vi "Main.vi"(11 "Module Admin":refnum<class "Delacor_lib_QMH_Cloneable Module Admin.lvclass">) -> ()   [LabVIEW 2020, in "NI DAQ.lvlib"]
doc: "This template is based off of the Queued Message Handler design pattern and the Queued Message Handler project template that ships with LabVIEW.\n\nThe main difference is that the queue is private to this module and communication between modules is performed via Broadcast and Request events.\n\nRequest events are wrapped in public API methods and are handled in the Event Handling Loop (EHL) of this VI. Any module can register for Broadcast events sent by this module. The EHL generates messages based on user interface actions.\n\nThe Message Handling Loop (MHL) processes messages generated by the EHL, or by other messages. The messages are string values, so new messages can be added easily to the Message Cases case structure in the MHL. Each message cluster can also provide an optional value for Message Data, which is a variant that can be converted to whatever message-specific data is required.\n_____\nBased on DQMH Project Template 6.1.0.94."
uses:
  NI DAQ.lvlib
  <vilib>/Delacor/Delacor QMH/Libraries/Cloneable Module Admin_class/Delacor_lib_QMH_Cloneable Module Admin.lvclass
  C:/Program Files (x86)/National Instruments/LabVIEW 2020/vi.lib/Delacor/Delacor QMH/Libraries/Module Admin_class/Delacor_lib_QMH_Module Admin.lvclass
  Module Data--cluster.ctl
  Support/Continuous aquisition params.ctl
  Support/Task list.ctl
  <vilib>/Delacor/Delacor QMH/Libraries/Message Queue_class/Delacor_lib_QMH_Message Queue.lvclass/Delacor_lib_QMH_Message Queue.ctl
  <vilib>/Delacor/Delacor QMH/Libraries/Cloneable Module Admin_class/Delacor_lib_QMH_Cloneable Module Admin.lvclass/Delacor_lib_QMH_Cloneable Module Admin.ctl
  Stop Argument--cluster.ctl
  <vilib>/Delacor/Delacor QMH/Libraries/Module Admin_class/Delacor_lib_QMH_Module Admin.lvclass/Delacor_lib_QMH_Module Admin.ctl
  Set device ID Argument--cluster.ctl
  Get channel list Argument--cluster.ctl
  Get channel list (Reply Payload)--cluster.ctl
  Create DO task Argument--cluster.ctl
  Create DO task (Reply Payload)--cluster.ctl
  Start task Argument--cluster.ctl
  Stop task Argument--cluster.ctl
  Write DO Argument--cluster.ctl
  Create DI channel Argument--cluster.ctl
  Read DI Argument--cluster.ctl
  Read DI (Reply Payload)--cluster.ctl
  Get task ref Argument--cluster.ctl
  Get task ref (Reply Payload)--cluster.ctl
  Create AI channel Argument--cluster.ctl
  Read AI Argument--cluster.ctl
  Read AI (Reply Payload)--cluster.ctl
  Create AO channel Argument--cluster.ctl
  AI config parameters--cluster.ctl
  Write AO Argument--cluster.ctl
  Validate connection Argument--cluster.ctl
  Validate connection (Reply Payload)--cluster.ctl
  Start continous acquisition Argument--cluster.ctl
  Stop continuous acquisition Argument--cluster.ctl
  <vilib>/Utility/miscctls.llb/LVPointTypeDef.ctl
  <vilib>/DAQmx/write.llb/DAQmx Write (Digital Bool 1Line 1Point).vi
  <vilib>/DAQmx/write.llb/DAQmx Write (Digital 1D Bool NChan 1Samp 1Line).vi
  <vilib>/DAQmx/read.llb/DAQmx Read (Digital 1D Bool 1Chan 1Samp).vi
  <vilib>/DAQmx/read.llb/DAQmx Read (Digital 1D Bool NChan 1Samp 1Line).vi
  <vilib>/DAQmx/write.llb/DAQmx Write (Analog DBL 1Chan 1Samp).vi
  <vilib>/DAQmx/write.llb/DAQmx Write (Analog 1D DBL NChan 1Samp).vi
  <vilib>/DAQmx/read.llb/DAQmx Read (Analog DBL 1Chan 1Samp).vi
  <vilib>/DAQmx/read.llb/DAQmx Read (Analog 1D DBL NChan 1Samp).vi
  <vilib>/Delacor/Delacor QMH/Libraries/Message Queue_class/Delacor_lib_QMH_Enqueue Message (Single).vi
  <vilib>/Delacor/Delacor QMH/Libraries/Cloneable Module Admin_class/Delacor_lib_QMH_Get Module ID.vi
  <vilib>/Delacor/Delacor QMH/Libraries/Module Admin_class/Delacor_lib_QMH_Get External Launch.vi
  <vilib>/DAQmx/write.llb/DAQmx Write (Digital 1D Bool 1Chan 1Samp).vi
  <vilib>/DAQmx/read.llb/DAQmx Read (Digital Bool 1Line 1Point).vi
  <vilib>/DAQmx/read.llb/DAQmx Read (Digital 1D U8 1Chan NSamp).vi
  <vilib>/DAQmx/miscellaneous.llb/DAQmx Fill In Error Info.vi
  <vilib>/Utility/error.llb/Error Cluster From Error Code.vi
  <vilib>/DAQmx/create/channels.llb/DAQmx Create Channel (DO-Digital Output).vi
  <vilib>/DAQmx/create/channels.llb/DAQmx Create Channel (DI-Digital Input).vi
  <vilib>/DAQmx/create/channels.llb/DAQmx Create Channel (AI-Voltage-Basic).vi
  <vilib>/DAQmx/create/channels.llb/DAQmx Create Channel (AO-Voltage-Basic).vi
  <vilib>/ErrorRing/Error Ring.xnode
  <vilib>/Delacor/Delacor QMH/Libraries/Message Queue_class/Delacor_lib_QMH_Message Queue.lvclass
  <resource>/objmgr/daqmx.rc
panel:
  out "error out":errorcluster
  out "Status":string
  in  "Simulate EHL Error":bool
  in  "Simulate MHL Error":bool
  # "Other QMH Modules communicate with this Module via its Public API (wrappers for its Request Events).\n\nThis Module communicates with other Modules via its Broadcast Events.\nAny module that wants to get these messages, just registers for this module's Broadcast events."
  # "This template is for the Delacor Modified Queued Message Handler design pattern.\n\nSee the block diagram for more information on how to use this template."
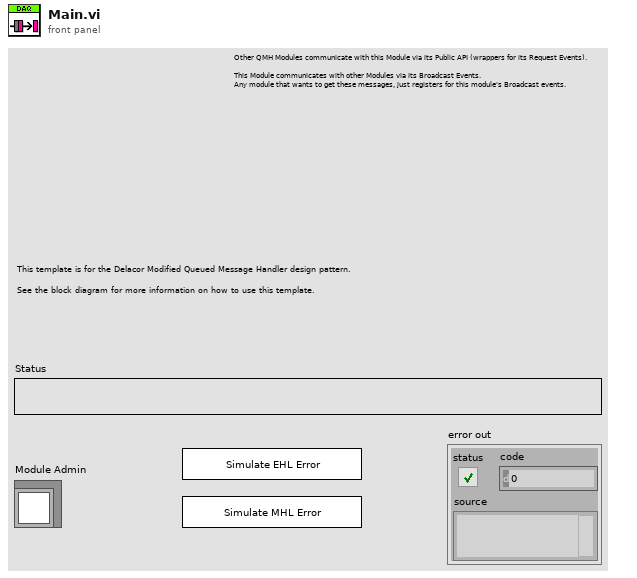
[diagram p1: front panel]
types:
  T1 = typedef "NI DAQ.lvlib/Request Events--cluster.ctl" = cluster{"Stop Module":refnum<user-event>, "Show Panel":refnum<user-event>, "Hide Panel":refnum<user-event>, "Show Diagram":refnum<user-event>, "Get Module Execution Status":refnum<user-event>, "Set device ID":refnum<user-event>, "Get channel list":refnum<user-event>, "Create DO task":refnum<user-event>, "Start task":refnum<user-event>, "Stop task":refnum<user-event>, "Write DO":refnum<user-event>, "Create DI channel":refnum<user-event>, "Read DI":refnum<user-event>, "Get task ref":refnum<user-event>, "Wake up HL":refnum<user-event>, "Sleep HL":refnum<user-event>, "Create AI channel":refnum<user-event>, "Read AI":refnum<user-event>, "Create AO channel":refnum<user-event>, "Write AO":refnum<user-event>, "Validate connection":refnum<user-event>, "Start continous acquisition":refnum<user-event>, "Stop continuous acquisition":refnum<user-event>}
  T2 = cluster{"Wake HL":refnum<user-event>, "Sleep HL":refnum<user-event>}
  T3 = typedef "NI DAQ.lvlib/Continuous aquisition params.ctl" = cluster{"Module ID":i32, "Task list":T4, "Timeout":i32, "Acq type":enum16{"Single", "Multiple"}, "Data in":variant, "DAQmx Task":refnum<k21>, "N samples":i32}
  T4 = typedef "NI DAQ.lvlib/Task list.ctl" = enum16{"All", "DO task", "DI task", "AO task", "AI task"}
  T5 = typedef "NI DAQ.lvlib/Module Data--cluster.ctl" = cluster{"Status":string, "DO task":refnum<k21>, "DI task":refnum<k21>, "AO task":refnum<k21>, "AI task":refnum<k21>, "Device name":tag}
  T6 = enum32{"invalid lock state", "Not Locked", "Locked (No Password)", "Password-protected"}
  T7 = typedef "NI DAQ.lvlib/Stop Argument--cluster.ctl" = cluster{"Module ID":i32, "Origin":string, "Exit via Stop Module Req?":bool, "Wait for Module to stop?":bool}
  T8 = typedef "NI DAQ.lvlib/Set device ID Argument--cluster.ctl" = cluster{"Module ID":i32, "Device ID":tag}
  T9 = typedef "NI DAQ.lvlib/Get channel list Argument--cluster.ctl" = cluster{"Module ID":i32, "Wait Notifier":refnum<notifier>, "wait for reply":bool}
  T10 = typedef "NI DAQ.lvlib/Create DO task Argument--cluster.ctl" = cluster{"Module ID":i32, "lines":tag, "Wait Notifier":refnum<notifier>, "wait for reply":bool, "Channel name":string}
  T11 = typedef "NI DAQ.lvlib/Start task Argument--cluster.ctl" = cluster{"Module ID":i32, "Boolean":bool}
  T12 = typedef "NI DAQ.lvlib/Stop task Argument--cluster.ctl" = cluster{"Module ID":i32, "Task list":T4}
  T13 = typedef "NI DAQ.lvlib/Write DO Argument--cluster.ctl" = cluster{"Module ID":i32, "Samples":enum16{"Single", "Multiple"}, "Data":bool[]}
  T14 = typedef "NI DAQ.lvlib/Create DI channel Argument--cluster.ctl" = cluster{"Module ID":i32, "Physical channel":string, "Channel name":string}
  T15 = typedef "NI DAQ.lvlib/Read DI Argument--cluster.ctl" = cluster{"Module ID":i32, "Samples":enum16{"Single", "Multiple"}, "Wait Notifier":refnum<notifier>, "wait for reply":bool}
  T16 = typedef "NI DAQ.lvlib/Get task ref Argument--cluster.ctl" = cluster{"Module ID":i32, "Task list":T4, "Wait Notifier":refnum<notifier>, "wait for reply":bool}
  T17 = typedef "NI DAQ.lvlib/Create AI channel Argument--cluster.ctl" = cluster{"Module ID":i32, "Physical channel":string, "Channel name":string, "Config params":cluster{"input terminal configuration":i32, "minimum value":dbl, "maximum value":dbl}}
  T18 = typedef "NI DAQ.lvlib/Read AI Argument--cluster.ctl" = cluster{"Module ID":i32, "Samples":enum16{"Single", "Multiple"}, "Wait Notifier":refnum<notifier>, "wait for reply":bool}
  T19 = typedef "NI DAQ.lvlib/Create AO channel Argument--cluster.ctl" = cluster{"Module ID":i32, "Physical channel":string, "Channel name":string, "Config params":T20}
  T20 = typedef "NI DAQ.lvlib/AI config parameters--cluster.ctl" = cluster{"Terminal configuration":i32, "min value":dbl, "max value":dbl}
  T21 = typedef "NI DAQ.lvlib/Write AO Argument--cluster.ctl" = cluster{"Module ID":i32, "Value(s)":dbl[], "Samples":enum16{"Single", "Multiple"}}
  T22 = typedef "NI DAQ.lvlib/Validate connection Argument--cluster.ctl" = cluster{"Module ID":i32, "Wait Notifier":refnum<notifier>, "wait for reply":bool}
  T23 = typedef "NI DAQ.lvlib/Start continous acquisition Argument--cluster.ctl" = cluster{"Module ID":i32, "Task list":T4, "Timeout":i32, "Acq type":enum16{"Single", "Multiple"}, "N samples":i32, "Data in":variant}
  T24 = typedef "NI DAQ.lvlib/Stop continuous acquisition Argument--cluster.ctl" = cluster{"Module ID":i32, "Boolean":bool}
  T25 = typedef "LVPointTypeDef.ctl" = cluster{"Horizontal":i16, "Vertical":i16}
  T26 = enum32{"Invalid", "Standard", "Closed", "Hidden", "Minimized", "Maximized"}
  T27 = typedef "NI DAQ.lvlib/Get channel list (Reply Payload)--cluster.ctl" = cluster{"Available channels":i32, "error":errorcluster}
  T28 = typedef "NI DAQ.lvlib/Create DO task (Reply Payload)--cluster.ctl" = cluster{"task out":refnum<k21>, "error":errorcluster}
  T29 = typedef "NI DAQ.lvlib/Read DI (Reply Payload)--cluster.ctl" = cluster{"Data":bool[], "error":errorcluster}
  T30 = typedef "NI DAQ.lvlib/Read AI (Reply Payload)--cluster.ctl" = cluster{"Data":dbl[], "error":errorcluster}
  T31 = typedef "NI DAQ.lvlib/Get task ref (Reply Payload)--cluster.ctl" = cluster{"DAQmx Task":refnum<k21>, "error":errorcluster}
  T32 = typedef "NI DAQ.lvlib/Validate connection (Reply Payload)--cluster.ctl" = cluster{"DevSerialNum":u32, "error":errorcluster}
  T33 = cluster{"input terminal configuration":i32, "minimum value":dbl, "maximum value":dbl}
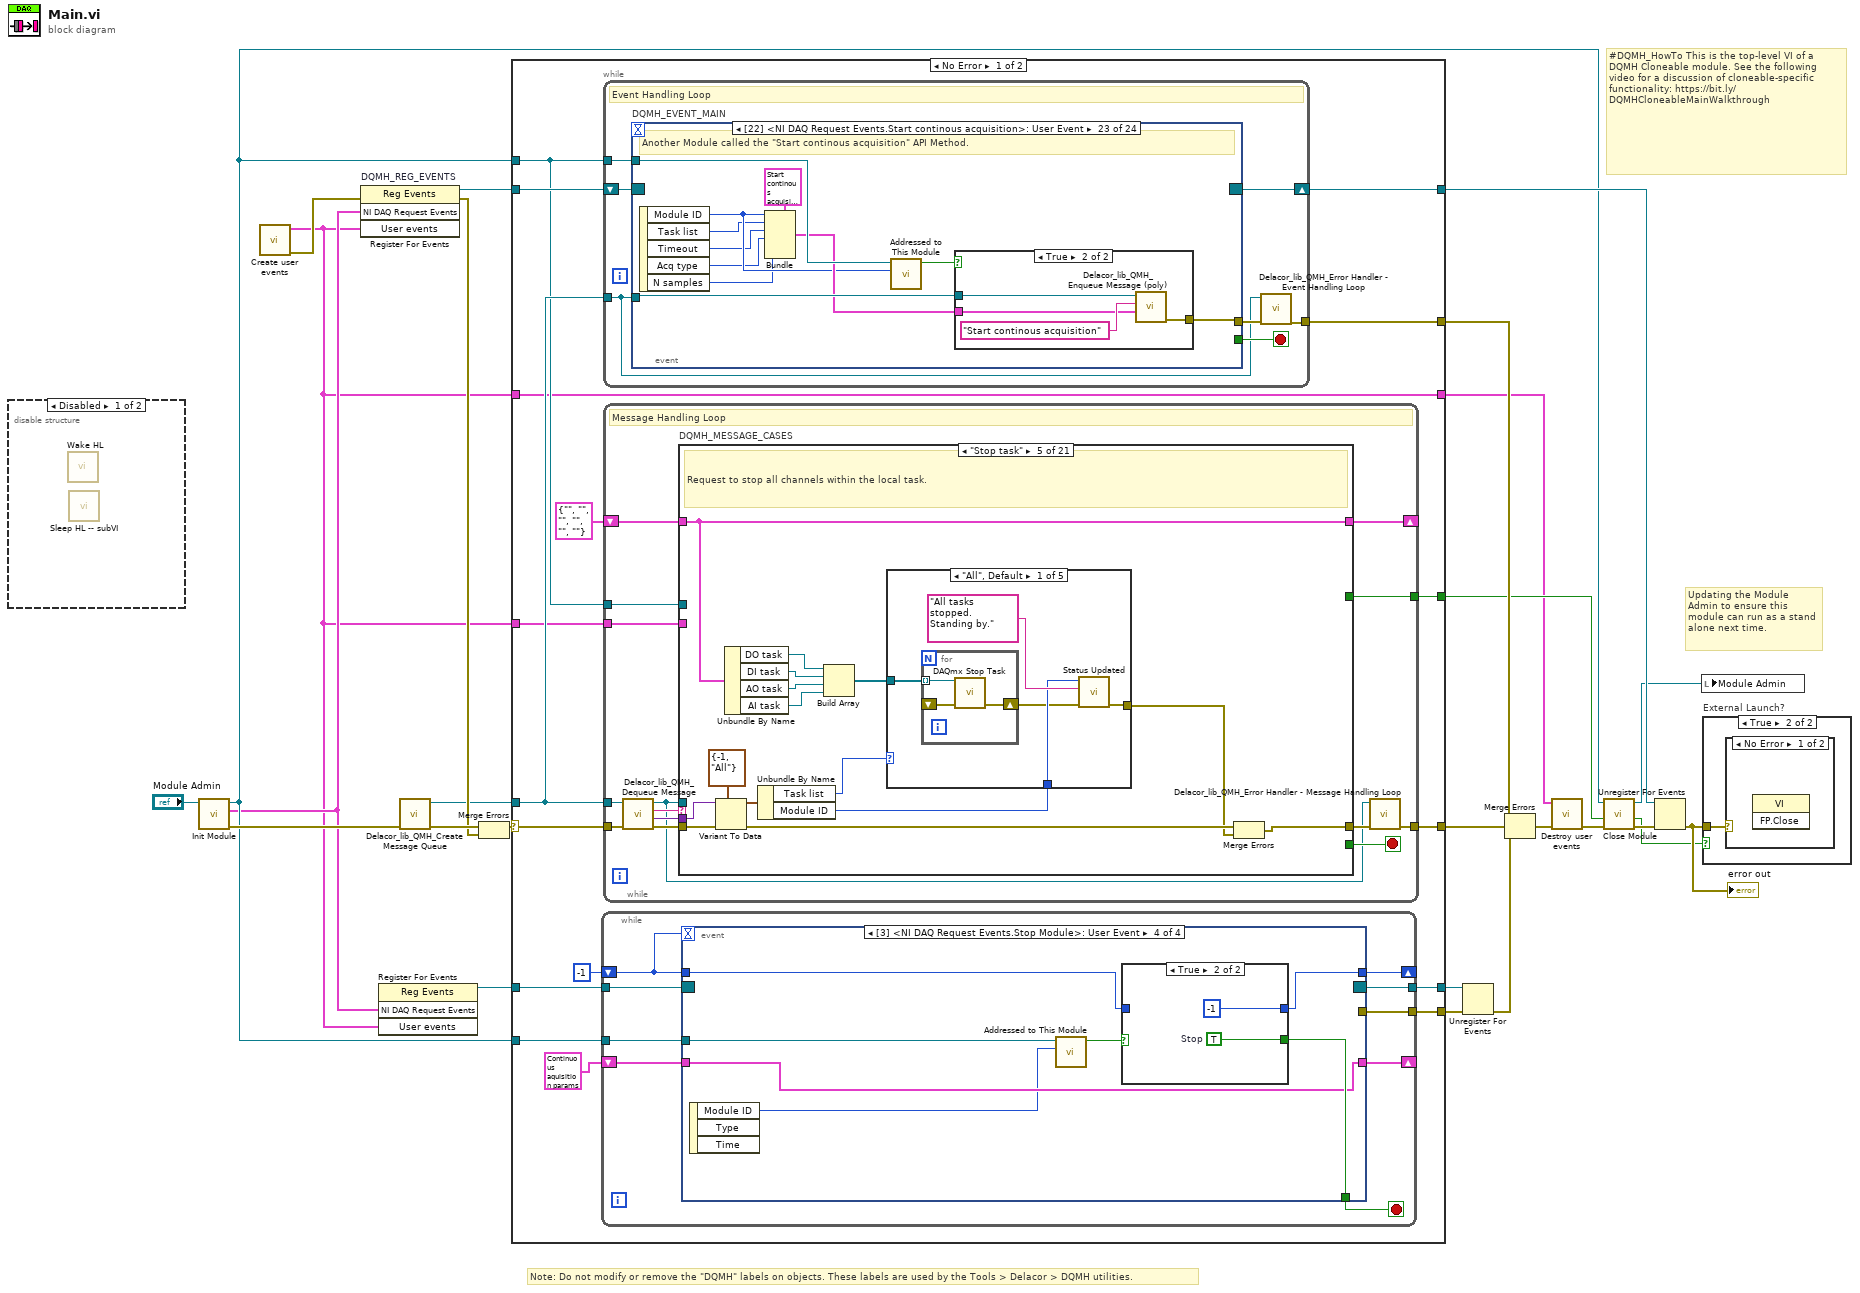
[diagram p0: block diagram]
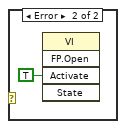
[diagram p4: hidden frame]
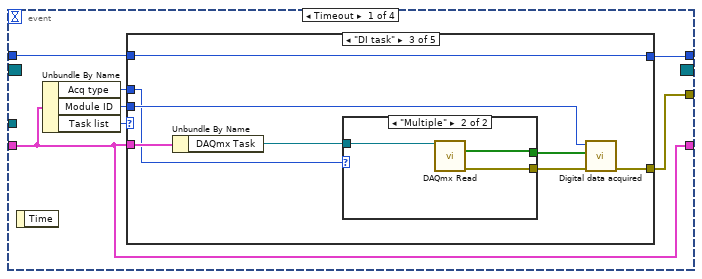
[diagram p5: hidden frame]
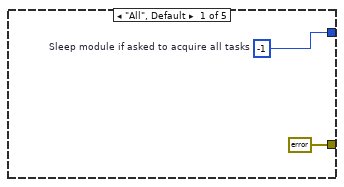
[diagram p6: hidden frame]
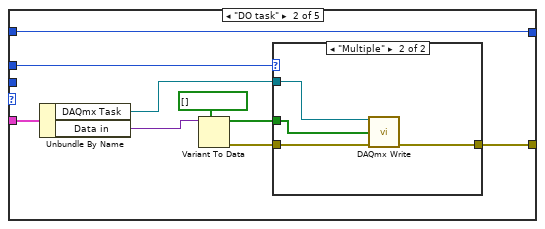
[diagram p7: hidden frame]
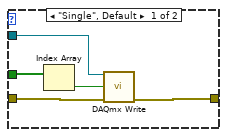
[diagram p8: hidden frame]
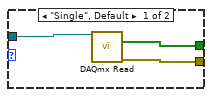
[diagram p9: hidden frame]
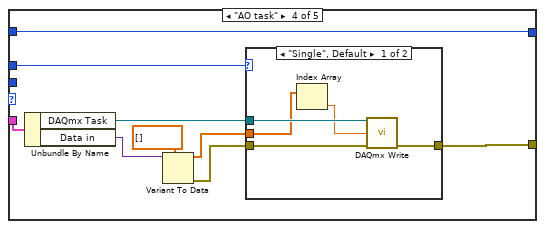
[diagram p10: hidden frame]
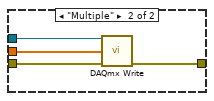
[diagram p11: hidden frame]
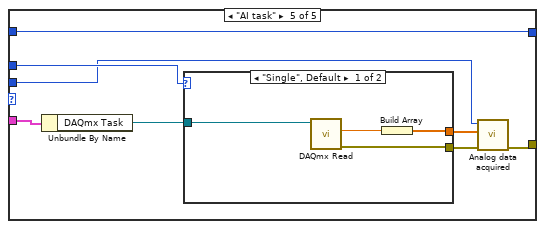
[diagram p12: hidden frame]
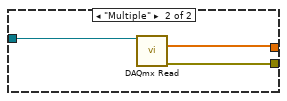
[diagram p13: hidden frame]
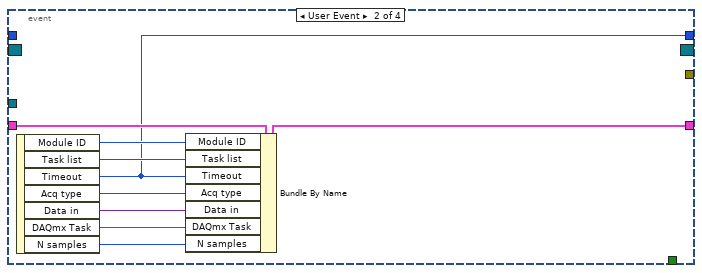
[diagram p14: hidden frame]
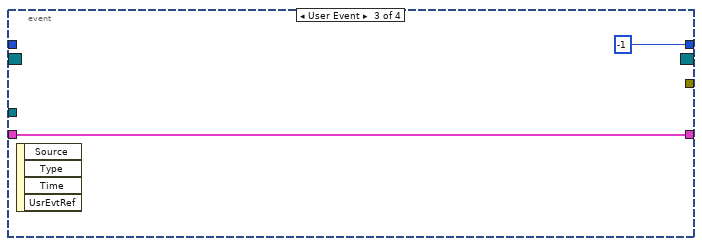
[diagram p15: hidden frame]
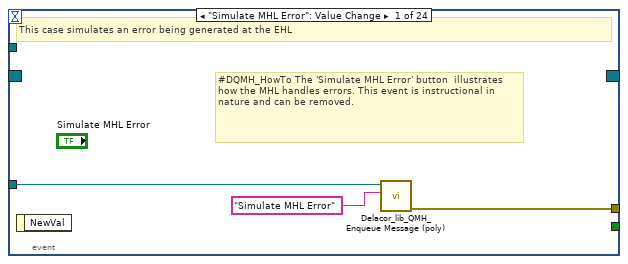
[diagram p17: hidden frame]
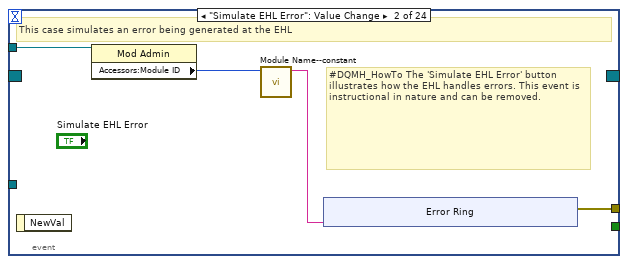
[diagram p18: hidden frame]
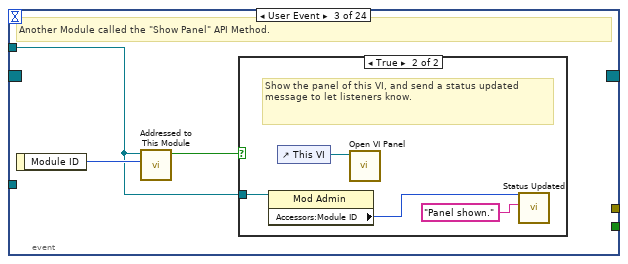
[diagram p19: hidden frame]
diagram:
  # "#DQMH_HowTo This is the top-level VI of a DQMH Cloneable module. See the following video for a discussion of cloneable-specific functionality: https://bit.ly/DQMHCloneableMainWalkthrough"
  # "Note: Do not modify or remove the \"DQMH\" labels on objects. These labels are used by the Tools > Delacor > DQMH utilities."
  # "Updating the Module Admin to ensure this module can run as a stand alone next time."
  n1 = disable-structure shown="Disabled" {
    frame Disabled {
      n2 = call "Wake HL.vi"() -> ()  [unwired: 11 in, 1 out]
      n3 = call "Sleep HL -- subVI.vi"() -> ()  [unwired: 11 in, 1 out]
    }
    frame Enabled {
    }
  }
  n4 = call "Init Module.vi"("Cloneable Module Admin in"="Module Admin") -> ("error out"=w24:errorcluster, "NI DAQ Request Events"=w8:T1, "Cloneable Module Admin out"=w10:refnum<class "Delacor_lib_QMH_Cloneable Module Admin.lvclass">)  [unwired: 8 in]
  n5 = call "Create user events.vi"() -> ("error out"=w9:errorcluster, "User events"=w2:T2)  [unwired: 10 in]
  n6 = register-events "DQMH_REG_EVENTS"(error in=w9, w8, w2) -> (reference out=w17:refnum<event-registration>, error out=w19:errorcluster)  [unwired: 1 in]
  n7 = register-events(w8, w2) -> (reference out=w11:refnum<event-registration>)  [unwired: 2 in, 1 out]
  n8 = call <vilib>:"Delacor_lib_QMH_Create Message Queue.vi"("error in"=w24) -> ("error out"=w21:errorcluster, "Message Queue"=w16:refnum<class "Delacor_lib_QMH_Message Queue.lvclass">)  [unwired: 9 in]
  n9 = Merge Errors(w21, w19) -> (w20:errorcluster)
  n10 = case shown="No Error" w20 {
    selector: w20 -> [w41 w944]
    tunnel: [w43 w943] -> w25
    tunnel: [w40 w951] -> w18
    tunnel: w17 -> [w38 w951]
    tunnel: w16 -> [w37 w942]
    tunnel: [w42 _] -> w26
    tunnel: w10 -> [w36 w947]
    tunnel: [w35 _] -> w13
    tunnel: w11 -> [w34 w941]
    tunnel: w10 -> [w32 _]
    tunnel: w2 -> [w31 w940]
    tunnel: [w31 w940] -> w7
    tunnel: [w30 w941] -> w4
    tunnel: w2 -> [w28 _]
    tunnel: [w27 _] -> w1
    frame No Error {
      n11 = while {
        tunnel: w34 -> [w52]
        shift-right: [w50] -> _
        shift-left: -1 -> [w46]
        shift-right: [w49] -> _
        shift-left: T3 {"Module ID"=0, "Task list"=enum."All", "Timeout"=0, "Acq type"=enum."Single", "Data in"=variant, "DAQmx Task"="", "N samples"=0} ("event data") -> [w48]
        tunnel: w32 -> [w47]
        tunnel: [w45] -> w30
        tunnel: [w44] -> w27
        stop <- w51 stop-if-true
        n12 = event shown="[3] <NI DAQ Request Events.Stop Module>: User Event" {
          selector: w52 -> [_ _ _ _]
          dyn-events: [_ _ _ _] -> w45
          timeout: w46 -> [_ _ _ _]
          tunnel: [_ _ _ w142] -> w51
          tunnel: [w59 w127 -1 ("Timeout") w143] -> w50
          tunnel: [w56 w128 w137 w139] -> w49
          tunnel: w48 -> [w56 w135 w137 w139]
          tunnel: w47 -> [_ _ _ w144]
          tunnel: w46 -> [w58 _ _ w141]
          tunnel: [w54 _ _ _] -> w44
          event Timeout {
            n13 = event-data() -> ()  [unwired: 1 in, 1 out]
            n14 = Unbundle By Name(w56) -> ("Acq type"=w53:enum16{"Single", "Multiple"}, "Module ID"=w55:i32, "Task list"=w57:T4)
            n15 = case shown="\"DI task\"" w57 {
              tunnel: [w61 w70 w87 w102 w119] -> w59
              tunnel: w58 -> [_ w70 w87 w102 w119]
              tunnel: w56 -> [_ w69 w86 w101 w117]
              tunnel: w55 -> [_ _ w82 _ w112]
              tunnel: [errorcluster {"status"=FALSE, "code"=0, "source"=""} ("error out") w63 w81 w94 w118] -> w54
              tunnel: w53 -> [_ w62 w80 w100 w116]
              frame "All", Default {
                w61 = -1  # Sleep module if asked to acquire all tasks
              }
              frame "DO task" {
                n16 = Unbundle By Name(w69) -> ("DAQmx Task"=w68:refnum<k21>, "Data in"=w66:variant)
                n17 = Variant To Data(type=bool[] [], Variant=w66) -> (data=w64:bool[], error out=w67:errorcluster)  [unwired: 1 in]
                n18 = case shown="\"Multiple\"" w62 {
                  tunnel: w68 -> [w75 w76]
                  tunnel: w67 -> [w74 w79]
                  tunnel: w64 -> [w72 w77]
                  tunnel: [w73 w78] -> w63
                  frame "Single", Default {
                    n19 = Index Array(array=w72) -> (element=w71:bool)  [unwired: 1 in]
                    n20 = call-poly <vilib>:"DAQmx Write.vi"("task/channels in"=w75, "data"=w71, "error in"=w74) -> ("error out"=w73:errorcluster)  [unwired: 10 in, 2 out]
                  }
                  frame "Multiple" {
                    n21 = call-poly <vilib>:"DAQmx Write.vi"("task/channels in"=w76, "data"=w77, "error in"=w79) -> ("error out"=w78:errorcluster)  [unwired: 10 in, 2 out]
                  }
                }
              }
              frame "DI task" {
                n22 = Unbundle By Name(w86) -> ("DAQmx Task"=w85:refnum<k21>)
                n23 = case shown="\"Multiple\"" w80 {
                  tunnel: w85 -> [w90 w91]
                  tunnel: [w89 w92] -> w84
                  tunnel: [w88 w93] -> w83
                  frame "Single", Default {
                    n24 = call-poly <vilib>:"DAQmx Read.vi"("task/channels in"=w90) -> ("data"=w89:bool[], "error out"=w88:errorcluster)  [unwired: 12 in, 1 out]
                  }
                  frame "Multiple" {
                    n25 = call-poly <vilib>:"DAQmx Read.vi"("task/channels in"=w91) -> ("data"=w92:bool[], "error out"=w93:errorcluster)  [unwired: 12 in, 1 out]
                  }
                }
                n26 = call "Digital data acquired.vi"("error in"=w83, "Data"=w84, "Module ID"=w82) -> ("error out"=w81:errorcluster)  [unwired: 8 in]
              }
              frame "AO task" {
                n27 = Unbundle By Name(w101) -> ("DAQmx Task"=w99:refnum<k21>, "Data in"=w98:variant)
                n28 = Variant To Data(type=dbl[] [], Variant=w98) -> (data=w95:dbl[], error out=w97:errorcluster)  [unwired: 1 in]
                n29 = case shown="\"Single\", Default" w100 {
                  tunnel: w99 -> [w107 w109]
                  tunnel: [w106 w111] -> w94
                  tunnel: w97 -> [w105 w110]
                  tunnel: w95 -> [w104 w108]
                  frame "Single", Default {
                    n30 = Index Array(array=w104) -> (element=w103:dbl)  [unwired: 1 in]
                    n31 = call-poly <vilib>:"DAQmx Write.vi"("task/channels in"=w107, "data"=w103, "error in"=w105) -> ("error out"=w106:errorcluster)  [unwired: 10 in, 2 out]
                  }
                  frame "Multiple" {
                    n32 = call-poly <vilib>:"DAQmx Write.vi"("task/channels in"=w109, "data"=w108, "error in"=w110) -> ("error out"=w111:errorcluster)  [unwired: 10 in, 2 out]
                  }
                }
              }
              frame "AI task" {
                n33 = Unbundle By Name(w117) -> ("DAQmx Task"=w115:refnum<k21>)
                n34 = case shown="\"Single\", Default" w116 {
                  tunnel: w115 -> [w123 w126]
                  tunnel: [w120 w125] -> w114
                  tunnel: [w122 w124] -> w113
                  frame "Single", Default {
                    n35 = call-poly <vilib>:"DAQmx Read.vi"("task/channels in"=w123) -> ("data"=w121:dbl, "error out"=w122:errorcluster)  [unwired: 12 in, 1 out]
                    n36 = Build Array(w121) -> (w120:dbl[])
                  }
                  frame "Multiple" {
                    n37 = call-poly <vilib>:"DAQmx Read.vi"("task/channels in"=w126) -> ("data"=w125:dbl[], "error out"=w124:errorcluster)  [unwired: 12 in, 1 out]
                  }
                }
                n38 = call "Analog data acquired.vi"("error in"=w113, "Data"=w114, "Module ID"=w112) -> ("error out"=w118:errorcluster)  [unwired: 8 in]
              }
            }
          }
          event User Event {
            n39 = event-data() -> ("Module ID"=w129:i32, "Task list"=w130:T4, "Timeout"=w127:i32, "Acq type"=w131:enum16{"Single", "Multiple"}, "Data in"=w132:variant, "DAQmx Task"=w133:refnum<k21>, "N samples"=w134:i32)  [unwired: 1 in]
            n40 = Bundle By Name(cluster=w135, "Module ID"=w129, "Task list"=w130, "Timeout"=w127, "Acq type"=w131, "Data in"=w132, "DAQmx Task"=w133, "N samples"=w134) -> (w128:T3)
          }
          event User Event {
            n41 = event-data() -> ()  [unwired: 1 in, 4 out]
          }
          event User Event {
            n42 = event-data() -> ("Module ID"=w138:i32)  [unwired: 1 in, 2 out]
            n43 = call "Addressed to This Module.vi"("Module ID from Argument"=w138, "Module Admin"=w144) -> ("Addressed to this instance?"=w140:bool)  [unwired: 8 in, 1 out]
            n44 = case shown="True" w140 {
              tunnel: [w145 -1] -> w143
              tunnel: [_ w146] -> w142
              tunnel: w141 -> [w145 _]
              frame False {
              }
              frame True {
                w146 = TRUE  # Stop
              }
            }
          }
        }
      }
      n45 = while {
        tunnel: w37 -> [w148]
        shift-right: [w151] -> w40
        shift-left: w38 -> [w152]
        tunnel: [w153] -> w42
        tunnel: w36 -> [w149]
        stop <- w150 stop-if-true
        # "Event Handling Loop"
        n46 = event "DQMH_EVENT_MAIN" shown="[22] <NI DAQ Request Events.Start continous acquisition>: User Event" {
          selector: w152 -> [_ _ _ _ _ _ _ _ _ _ _ _ _ _ _ _ _ _ _ _ _ _ _ _]
          dyn-events: [_ _ _ _ _ _ _ _ _ _ _ _ _ _ _ _ _ _ _ _ _ _ _ _] -> w151
          timeout: _ -> [_ _ _ _ _ _ _ _ _ _ _ _ _ _ _ _ _ _ _ _ _ _ _ _]
          tunnel: [_ _ _ _ _ _ w209 _ _ _ _ _ _ _ _ _ _ _ _ _ _ _ _ _] -> w150
          tunnel: w148 -> [w156 _ _ _ _ _ w212 w228 w244 w257 w272 w284 w296 w309 w322 w336 w350 w364 w378 w392 w405 w418 w433 w445]
          tunnel: [w157 w161 _ _ w186 _ w213 w231 w237 w251 w263 w277 w290 w302 w314 w327 w341 w357 w369 w384 w398 w412 w423 w438] -> w154
          tunnel: w149 -> [_ w160 w169 w176 w184 w190 w211 w229 w242 w255 w270 w282 w294 w307 w320 w334 w348 w362 w376 w390 w403 w416 w431 w443]
          event "Simulate MHL Error": Value Change {
            # "#DQMH_HowTo The 'Simulate MHL Error' button  illustrates how the MHL handles errors. This event is instructional in nature and can be removed."
            # "This case simulates an error being generated at the EHL"
            n47 = event-data() -> ()  [unwired: 1 in, 1 out]
            n48 = call-poly <vilib>:"Delacor_lib_QMH_Enqueue Message (poly).vi"("Message"="Simulate MHL Error", "Message Queue in"=w156) -> ("error out"=w157:errorcluster)  [unwired: 8 in, 1 out]
          }
          event "Simulate EHL Error": Value Change {
            # "#DQMH_HowTo The 'Simulate EHL Error' button  illustrates how the EHL handles errors. This event is instructional in nature and can be removed."
            # "This case simulates an error being generated at the EHL"
            n49 = event-data() -> ()  [unwired: 1 in, 1 out]
            n50 = property class="Mod Admin"(reference=w160) -> ("Accessors:Module ID"=w159:i32)  [unwired: 1 in, 2 out]
            n51 = call "Module Name--constant.vi"("Module ID"=w159) -> ("Module Name"=w158:string)  [unwired: 10 in]
            n52 = xnode "Error Ring"("parameter 0"=w158) -> ("error out"=w161:errorcluster)
          }
          event User Event {
            # "Another Module called the \"Show Panel\" API Method."
            n53 = event-data() -> ("Module ID"=w170:i32)  [unwired: 1 in]
            n54 = call "Addressed to This Module.vi"("Module ID from Argument"=w170, "Module Admin"=w169) -> ("Addressed to this instance?"=w171:bool)  [unwired: 8 in, 1 out]
            n55 = case shown="True" w171 {
              tunnel: w169 -> [_ w173]
              frame False {
              }
              frame True {
                # "Show the panel of this VI, and send a status updated message to let listeners know."
                n56 = property class="Mod Admin"(reference=w173) -> ("Accessors:Module ID"=w172:i32)  [unwired: 1 in, 2 out]
                n57 = control-ref of="This VI"() -> (w175:refnum<vi>)
                n58 = call "Open VI Panel.vi"("VI"=w175) -> ()  [unwired: 10 in, 1 out]
                n59 = call "Status Updated.vi"("Status"="Panel shown." ("format string"), "Module ID"=w172) -> ()  [unwired: 9 in, 1 out]
              }
            }
          }
          event User Event {
            # "Another Module called the \"Hide Panel\" API Method."
            n60 = event-data() -> ("Module ID"=w177:i32)  [unwired: 1 in]
            n61 = call "Addressed to This Module.vi"("Module ID from Argument"=w177, "Module Admin"=w176) -> ("Addressed to this instance?"=w178:bool)  [unwired: 8 in, 1 out]
            n62 = case shown="True" w178 {
              tunnel: w176 -> [_ w180]
              frame False {
              }
              frame True {
                # "Hide the panel of this VI, and send a status updated message to let listeners know."
                n63 = property class="Mod Admin"(reference=w180) -> ("Accessors:Module ID"=w179:i32)  [unwired: 1 in, 2 out]
                n64 = control-ref of="This VI"() -> (w182:refnum<vi>)
                n65 = call "Hide VI Panel.vi"("VI"=w182) -> ()  [unwired: 10 in, 1 out]
                n66 = call "Status Updated.vi"("Status"="Panel hidden." ("format string"), "Module ID"=w179) -> ()  [unwired: 9 in, 1 out]
              }
            }
          }
          event User Event {
            # "For cloneable running as singleton, broadcast that the module is running."
            n67 = event-data() -> ("Module ID"=w183:i32)  [unwired: 1 in]
            n68 = call "Addressed to This Module.vi"("Module ID from Argument"=w183, "Module Admin"=w184) -> ("Addressed to this instance?"=w185:bool)  [unwired: 8 in, 1 out]
            n69 = case shown="True" w185 {
              tunnel: [_ w189] -> w186
              tunnel: w183 -> [_ w188]
              frame False {
              }
              frame True {
                n70 = call "Update Module Execution Status.vi"("Running?"=TRUE, "Module ID"=w188) -> ("error out"=w189:errorcluster)  [unwired: 9 in]
              }
            }
          }
          event User Event {
            # "Another Module called the \"Show Diagram\" API Method. This event is used for debugging."
            n71 = event-data() -> ("Module ID"=w191:i32)  [unwired: 1 in]
            n72 = call "Addressed to This Module.vi"("Module ID from Argument"=w191, "Module Admin"=w190) -> ("Addressed to this instance?"=w192:bool)  [unwired: 8 in, 1 out]
            n73 = case shown="True" w192 {
              tunnel: w190 -> [_ w193]
              frame False {
              }
              frame True {
                n74 = disable-structure shown="RUN_TIME_ENGINE==False" {
                  disable-tunnel: w193 -> [w194 _]
                  frame condition #0 (active) {
                    # "functionality not available in exe"
                    n75 = invoke class="VI" method="Lock State.Get"() -> (error out=w200:errorcluster, "Get Lock State"=w199:T6, "pwd in cache"=w196:bool)  [unwired: 4 in, 1 out]
                    n76 = Equal?(x=T6."Password-protected", y=w199) -> (x = y?=w197:bool)
                    n77 = Compound Arithmetic op=AND(w197, invert w196) -> (w195:bool)
                    n78 = case shown="False" w195 {
                      tunnel: w200 -> [w205 _]
                      tunnel: w194 -> [w202 _]
                      frame False {
                        n79 = property class="Mod Admin"(reference=w202) -> ("Accessors:Module ID"=w201:i32)  [unwired: 1 in, 2 out]
                        n80 = property class="VI"(error in=w205, "BDWin.Open"=TRUE ("Block Diagram Window:Open")) -> ()  [unwired: 1 in, 2 out]
                        n81 = call "Status Updated.vi"("Status"="Block Diagram shown." ("format string"), "Module ID"=w201) -> ()  [unwired: 9 in, 1 out]
                      }
                      frame True {
                        # "Password-protected VI, and the password is not in the cache. Do not show the diagram."
                      }
                    }
                  }
                  frame condition #1 {
                  }
                }
              }
            }
          }
          event User Event {
            # "Another Module called the \"Stop Module\" API Method  or the Message Handling Loop below."
            n82 = event-data() -> ("Module ID"=w207:i32, "Wait for Module to stop?"=w208:bool, "Origin"=w206:string)  [unwired: 1 in]
            n83 = call "Addressed to This Module.vi"("Module ID from Argument"=w207, "Module Admin"=w211) -> ("Addressed to this instance?"=w210:bool)  [unwired: 8 in, 1 out]
            n84 = case shown="True" w210 {
              tunnel: [_ w225] -> w213
              tunnel: w212 -> [_ w221]
              tunnel: [_ TRUE] -> w209
              tunnel: w208 -> [_ w216]
              tunnel: w207 -> [_ w218]
              tunnel: w206 -> [_ w214]
              frame False {
              }
              frame True {
                # "The event can get fired from the Exit message. The queue gets destroyed there. In this case, the Enqueue VI will return error 1. It is safe to ignore, because the module is already exiting."
                n85 = local write "Status"(w214) -> ()
                n86 = Bundle By Name(cluster=T7 {"Module ID"=-1, "Origin"="", "Exit via Stop Module Req?"=FALSE, "Wait for Module to stop?"=FALSE} ("Stop Argument"), "Module ID"=w218, "Exit via Stop Module Req?"=TRUE, "Wait for Module to stop?"=w216) -> (w215:T7)
                n87 = call-poly <vilib>:"Delacor_lib_QMH_Enqueue Message (poly).vi"("Priority Message? (F)"=TRUE, "Message Data"=w215, "Message"="Exit", "Message Queue in"=w221) -> ("error out"=w226:errorcluster)  [unwired: 6 in, 1 out]
                n88 = call <vilib>:"Clear Errors.vi"("error in (no error)"=w226, "specific error code to clear (0: all)"=1) -> ("error out"=w225:errorcluster)  [unwired: 4 in, 1 out]
              }
            }
          }
          event Panel Close? {
            w230 = TRUE  # Discard the event, the MHL is responsible for closing and stopping this VI.
            # "Hide the panel or send the 'Exit' message if the user clicks the 'X' on the module main VI panel."
            n89 = event-data() -> ()  [unwired: 1 in, 1 out]
            n90 = property class="Mod Admin"(reference=w229) -> ("Accessors:External Launch"=w227:bool)  [unwired: 1 in, 2 out]
            n91 = case shown="True" w227 {
              tunnel: w228 -> [_ w235]
              tunnel: [_ w236] -> w231
              frame True {
                # "If externally launched, clicking the 'X' hides the panel, but doesn't close it."
                n92 = control-ref of="This VI"() -> (w232:refnum<vi>)
                n93 = call "Hide VI Panel.vi"("VI"=w232) -> ()  [unwired: 10 in, 1 out]
              }
              frame False {
                # "If run as a stand-alone VI, clicking the panel 'X' stops the VI."
                n94 = call-poly <vilib>:"Delacor_lib_QMH_Enqueue Message (poly).vi"("Priority Message? (F)"=TRUE, "Message"="Exit", "Message Queue in"=w235) -> ("error out"=w236:errorcluster)  [unwired: 7 in, 1 out]
              }
            }
            n95 = event-data("Discard?"=w230) -> ()  [unwired: 1 in, 1 out]
          }
          event User Event {
            # "Another Module called the \"Set device ID\" API Method."
            n96 = event-data() -> ("Module ID"=w239:i32, "Device ID"=w238:tag)  [unwired: 1 in]
            n97 = Bundle(cluster=T8 {"Module ID"=-1, "Device ID"=""} ("Set device ID Argument"), "Module ID"=w239, "Device ID"=w238) -> (w240:T8)
            n98 = call "Addressed to This Module.vi"("Module ID from Argument"=w239, "Module Admin"=w242) -> ("Addressed to this instance?"=w243:bool)  [unwired: 8 in, 1 out]
            n99 = case shown="True" w243 {
              tunnel: w244 -> [_ w248]
              tunnel: w240 -> [_ w246]
              tunnel: [_ w245] -> w237
              frame False {
              }
              frame True {
                n100 = call-poly <vilib>:"Delacor_lib_QMH_Enqueue Message (poly).vi"("Message Data"=w246, "Message"="Set device ID", "Message Queue in"=w248) -> ("error out"=w245:errorcluster)  [unwired: 7 in, 1 out]
              }
            }
          }
          event User Event {
            # "Another Module called the \"Get channel list\" API Method."
            n101 = event-data() -> ("Module ID"=w252:i32, "Wait Notifier"=w250:refnum<notifier>, "wait for reply"=w249:bool)  [unwired: 1 in]
            n102 = Bundle(cluster=T9 {"Module ID"=-1, "Wait Notifier"=refnum, "wait for reply"=FALSE} ("Get channel list Argument"), "Module ID"=w252, "Wait Notifier"=w250, "wait for reply"=w249) -> (w253:T9)
            n103 = call "Addressed to This Module.vi"("Module ID from Argument"=w252, "Module Admin"=w255) -> ("Addressed to this instance?"=w256:bool)  [unwired: 8 in, 1 out]
            n104 = case shown="True" w256 {
              tunnel: w257 -> [_ w261]
              tunnel: w253 -> [_ w259]
              tunnel: [_ w258] -> w251
              frame False {
              }
              frame True {
                n105 = call-poly <vilib>:"Delacor_lib_QMH_Enqueue Message (poly).vi"("Message Data"=w259, "Message"="Get channel list", "Message Queue in"=w261) -> ("error out"=w258:errorcluster)  [unwired: 7 in, 1 out]
              }
            }
          }
          event User Event {
            # "Another Module called the \"Create DO task\" API Method."
            n106 = event-data() -> ("Module ID"=w267:i32, "lines"=w266:tag, "Wait Notifier"=w265:refnum<notifier>, "wait for reply"=w264:bool, "Channel name"=w262:string)  [unwired: 1 in]
            n107 = Bundle(cluster=T10 {"Module ID"=-1, "lines"="", "Wait Notifier"=refnum, "wait for reply"=FALSE, "Channel name"=""} ("Create DO task Argument"), "Module ID"=w267, "lines"=w266, "Wait Notifier"=w265, "wait for reply"=w264, "Channel name"=w262) -> (w268:T10)
            n108 = call "Addressed to This Module.vi"("Module ID from Argument"=w267, "Module Admin"=w270) -> ("Addressed to this instance?"=w271:bool)  [unwired: 8 in, 1 out]
            n109 = case shown="True" w271 {
              tunnel: w272 -> [_ w276]
              tunnel: w268 -> [_ w274]
              tunnel: [_ w273] -> w263
              frame False {
              }
              frame True {
                n110 = call-poly <vilib>:"Delacor_lib_QMH_Enqueue Message (poly).vi"("Message Data"=w274, "Message"="Create DO channel", "Message Queue in"=w276) -> ("error out"=w273:errorcluster)  [unwired: 7 in, 1 out]
              }
            }
          }
          event User Event {
            # "Another Module called the \"Start task\" API Method."
            n111 = event-data() -> ("Module ID"=w279:i32, "Boolean"=w278:bool)  [unwired: 1 in]
            n112 = Bundle(cluster=T11 {"Module ID"=-1, "Boolean"=FALSE} ("Start task Argument"), "Module ID"=w279, "Boolean"=w278) -> (w280:T11)
            n113 = call "Addressed to This Module.vi"("Module ID from Argument"=w279, "Module Admin"=w282) -> ("Addressed to this instance?"=w283:bool)  [unwired: 8 in, 1 out]
            n114 = case shown="True" w283 {
              tunnel: w284 -> [_ w288]
              tunnel: w280 -> [_ w286]
              tunnel: [_ w285] -> w277
              frame False {
              }
              frame True {
                n115 = call-poly <vilib>:"Delacor_lib_QMH_Enqueue Message (poly).vi"("Message Data"=w286, "Message"="Start task", "Message Queue in"=w288) -> ("error out"=w285:errorcluster)  [unwired: 7 in, 1 out]
              }
            }
          }
          event User Event {
            # "Another Module called the \"Stop task\" API Method."
            n116 = event-data() -> ("Module ID"=w291:i32, "Task list"=w289:T4)  [unwired: 1 in]
            n117 = Bundle(cluster=T12 {"Module ID"=-1, "Task list"=enum."All"} ("Stop task Argument"), "Module ID"=w291, "Task list"=w289) -> (w292:T12)
            n118 = call "Addressed to This Module.vi"("Module ID from Argument"=w291, "Module Admin"=w294) -> ("Addressed to this instance?"=w295:bool)  [unwired: 8 in, 1 out]
            n119 = case shown="True" w295 {
              tunnel: w296 -> [_ w300]
              tunnel: w292 -> [_ w298]
              tunnel: [_ w297] -> w290
              frame False {
              }
              frame True {
                n120 = call-poly <vilib>:"Delacor_lib_QMH_Enqueue Message (poly).vi"("Message Data"=w298, "Message"="Stop task", "Message Queue in"=w300) -> ("error out"=w297:errorcluster)  [unwired: 7 in, 1 out]
              }
            }
          }
          event User Event {
            # "Another Module called the \"Write DO\" API Method."
            n121 = event-data() -> ("Module ID"=w304:i32, "Samples"=w303:enum16{"Single", "Multiple"}, "Data"=w301:bool[])  [unwired: 1 in]
            n122 = Bundle(cluster=T13 {"Module ID"=-1, "Samples"=enum."Single", "Data"=[]} ("Write DO Argument"), "Module ID"=w304, "Samples"=w303, "Data"=w301) -> (w305:T13)
            n123 = call "Addressed to This Module.vi"("Module ID from Argument"=w304, "Module Admin"=w307) -> ("Addressed to this instance?"=w308:bool)  [unwired: 8 in, 1 out]
            n124 = case shown="True" w308 {
              tunnel: w309 -> [_ w313]
              tunnel: w305 -> [_ w311]
              tunnel: [_ w310] -> w302
              frame False {
              }
              frame True {
                n125 = call-poly <vilib>:"Delacor_lib_QMH_Enqueue Message (poly).vi"("Message Data"=w311, "Message"="Write DO", "Message Queue in"=w313) -> ("error out"=w310:errorcluster)  [unwired: 7 in, 1 out]
              }
            }
          }
          event User Event {
            # "Another Module called the \"Create DI channel\" API Method."
            n126 = event-data() -> ("Module ID"=w317:i32, "Physical channel"=w316:string, "Channel name"=w315:string)  [unwired: 1 in]
            n127 = Bundle(cluster=T14 {"Module ID"=-1, "Physical channel"="", "Channel name"=""} ("Create DI channel Argument"), "Module ID"=w317, "Physical channel"=w316, "Channel name"=w315) -> (w318:T14)
            n128 = call "Addressed to This Module.vi"("Module ID from Argument"=w317, "Module Admin"=w320) -> ("Addressed to this instance?"=w321:bool)  [unwired: 8 in, 1 out]
            n129 = case shown="True" w321 {
              tunnel: w322 -> [_ w326]
              tunnel: w318 -> [_ w324]
              tunnel: [_ w323] -> w314
              frame False {
              }
              frame True {
                n130 = call-poly <vilib>:"Delacor_lib_QMH_Enqueue Message (poly).vi"("Message Data"=w324, "Message"="Create DI channel", "Message Queue in"=w326) -> ("error out"=w323:errorcluster)  [unwired: 7 in, 1 out]
              }
            }
          }
          event User Event {
            # "Another Module called the \"Read DI\" API Method."
            n131 = event-data() -> ("Module ID"=w331:i32, "Samples"=w330:enum16{"Single", "Multiple"}, "Wait Notifier"=w329:refnum<notifier>, "wait for reply"=w328:bool)  [unwired: 1 in]
            n132 = Bundle(cluster=T15 {"Module ID"=-1, "Samples"=enum."Single", "Wait Notifier"=refnum, "wait for reply"=FALSE} ("Read DI Argument"), "Module ID"=w331, "Samples"=w330, "Wait Notifier"=w329, "wait for reply"=w328) -> (w332:T15)
            n133 = call "Addressed to This Module.vi"("Module ID from Argument"=w331, "Module Admin"=w334) -> ("Addressed to this instance?"=w335:bool)  [unwired: 8 in, 1 out]
            n134 = case shown="True" w335 {
              tunnel: w336 -> [_ w340]
              tunnel: w332 -> [_ w338]
              tunnel: [_ w337] -> w327
              frame False {
              }
              frame True {
                n135 = call-poly <vilib>:"Delacor_lib_QMH_Enqueue Message (poly).vi"("Message Data"=w338, "Message"="Read DI", "Message Queue in"=w340) -> ("error out"=w337:errorcluster)  [unwired: 7 in, 1 out]
              }
            }
          }
          event User Event {
            # "Another Module called the \"Get task ref\" API Method."
            n136 = event-data() -> ("Module ID"=w345:i32, "Task list"=w344:T4, "Wait Notifier"=w343:refnum<notifier>, "wait for reply"=w342:bool)  [unwired: 1 in]
            n137 = Bundle(cluster=T16 {"Module ID"=-1, "Task list"=enum."All", "Wait Notifier"=refnum, "wait for reply"=FALSE} ("Get task ref Argument"), "Module ID"=w345, "Task list"=w344, "Wait Notifier"=w343, "wait for reply"=w342) -> (w346:T16)
            n138 = call "Addressed to This Module.vi"("Module ID from Argument"=w345, "Module Admin"=w348) -> ("Addressed to this instance?"=w349:bool)  [unwired: 8 in, 1 out]
            n139 = case shown="True" w349 {
              tunnel: w350 -> [_ w354]
              tunnel: w346 -> [_ w352]
              tunnel: [_ w351] -> w341
              frame False {
              }
              frame True {
                n140 = call-poly <vilib>:"Delacor_lib_QMH_Enqueue Message (poly).vi"("Message Data"=w352, "Message"="Get task ref", "Message Queue in"=w354) -> ("error out"=w351:errorcluster)  [unwired: 7 in, 1 out]
              }
            }
          }
          event User Event {
            # "Another Module called the \"Create AI channel\" API Method."
            n141 = event-data() -> ("Module ID"=w359:i32, "Physical channel"=w358:string, "Channel name"=w356:string, "Config params"=w355:T33)  [unwired: 1 in]
            n142 = Bundle(cluster=T17 {"Module ID"=-1, "Physical channel"="", "Channel name"="", "Config params"={"input terminal configuration"=-1, "minimum value"=-5.0, "maximum value"=5.0}} ("Create AI channel Argument"), "Module ID"=w359, "Physical channel"=w358, "Channel name"=w356, "Config params"=w355) -> (w360:T17)
            n143 = call "Addressed to This Module.vi"("Module ID from Argument"=w359, "Module Admin"=w362) -> ("Addressed to this instance?"=w363:bool)  [unwired: 8 in, 1 out]
            n144 = case shown="True" w363 {
              tunnel: w364 -> [_ w368]
              tunnel: w360 -> [_ w366]
              tunnel: [_ w365] -> w357
              frame False {
              }
              frame True {
                n145 = call-poly <vilib>:"Delacor_lib_QMH_Enqueue Message (poly).vi"("Message Data"=w366, "Message"="Create AI channel", "Message Queue in"=w368) -> ("error out"=w365:errorcluster)  [unwired: 7 in, 1 out]
              }
            }
          }
          event User Event {
            # "Another Module called the \"Read AI\" API Method."
            n146 = event-data() -> ("Module ID"=w373:i32, "Samples"=w372:enum16{"Single", "Multiple"}, "Wait Notifier"=w371:refnum<notifier>, "wait for reply"=w370:bool)  [unwired: 1 in]
            n147 = Bundle(cluster=T18 {"Module ID"=-1, "Samples"=enum."Single", "Wait Notifier"=refnum, "wait for reply"=FALSE} ("Read AI Argument"), "Module ID"=w373, "Samples"=w372, "Wait Notifier"=w371, "wait for reply"=w370) -> (w374:T18)
            n148 = call "Addressed to This Module.vi"("Module ID from Argument"=w373, "Module Admin"=w376) -> ("Addressed to this instance?"=w377:bool)  [unwired: 8 in, 1 out]
            n149 = case shown="True" w377 {
              tunnel: w378 -> [_ w382]
              tunnel: w374 -> [_ w380]
              tunnel: [_ w379] -> w369
              frame False {
              }
              frame True {
                n150 = call-poly <vilib>:"Delacor_lib_QMH_Enqueue Message (poly).vi"("Message Data"=w380, "Message"="Read AI", "Message Queue in"=w382) -> ("error out"=w379:errorcluster)  [unwired: 7 in, 1 out]
              }
            }
          }
          event User Event {
            # "Another Module called the \"Create AO channel\" API Method."
            n151 = event-data() -> ("Module ID"=w387:i32, "Physical channel"=w386:string, "Channel name"=w385:string, "Config params"=w383:T20)  [unwired: 1 in]
            n152 = Bundle(cluster=T19 {"Module ID"=-1, "Physical channel"="", "Channel name"="", "Config params"={"Terminal configuration"=-1, "min value"=-5.0, "max value"=5.0}} ("Create AO channel Argument"), "Module ID"=w387, "Physical channel"=w386, "Channel name"=w385, "Config params"=w383) -> (w388:T19)
            n153 = call "Addressed to This Module.vi"("Module ID from Argument"=w387, "Module Admin"=w390) -> ("Addressed to this instance?"=w391:bool)  [unwired: 8 in, 1 out]
            n154 = case shown="True" w391 {
              tunnel: w392 -> [_ w396]
              tunnel: w388 -> [_ w394]
              tunnel: [_ w393] -> w384
              frame False {
              }
              frame True {
                n155 = call-poly <vilib>:"Delacor_lib_QMH_Enqueue Message (poly).vi"("Message Data"=w394, "Message"="Create AO channel", "Message Queue in"=w396) -> ("error out"=w393:errorcluster)  [unwired: 7 in, 1 out]
              }
            }
          }
          event User Event {
            # "Another Module called the \"Write AO\" API Method."
            n156 = event-data() -> ("Module ID"=w400:i32, "Value(s)"=w399:dbl[], "Samples"=w397:enum16{"Single", "Multiple"})  [unwired: 1 in]
            n157 = Bundle(cluster=T21 {"Module ID"=-1, "Value(s)"=[], "Samples"=enum."Single"} ("Write AO Argument"), "Module ID"=w400, "Value(s)"=w399, "Samples"=w397) -> (w401:T21)
            n158 = call "Addressed to This Module.vi"("Module ID from Argument"=w400, "Module Admin"=w403) -> ("Addressed to this instance?"=w404:bool)  [unwired: 8 in, 1 out]
            n159 = case shown="True" w404 {
              tunnel: w405 -> [_ w409]
              tunnel: w401 -> [_ w407]
              tunnel: [_ w406] -> w398
              frame False {
              }
              frame True {
                n160 = call-poly <vilib>:"Delacor_lib_QMH_Enqueue Message (poly).vi"("Message Data"=w407, "Message"="Write AO", "Message Queue in"=w409) -> ("error out"=w406:errorcluster)  [unwired: 7 in, 1 out]
              }
            }
          }
          event User Event {
            # "Another Module called the \"Validate connection\" API Method."
            n161 = event-data() -> ("Module ID"=w413:i32, "Wait Notifier"=w411:refnum<notifier>, "wait for reply"=w410:bool)  [unwired: 1 in]
            n162 = Bundle(cluster=T22 {"Module ID"=-1, "Wait Notifier"=refnum, "wait for reply"=FALSE} ("Validate connection Argument"), "Module ID"=w413, "Wait Notifier"=w411, "wait for reply"=w410) -> (w414:T22)
            n163 = call "Addressed to This Module.vi"("Module ID from Argument"=w413, "Module Admin"=w416) -> ("Addressed to this instance?"=w417:bool)  [unwired: 8 in, 1 out]
            n164 = case shown="True" w417 {
              tunnel: w418 -> [_ w422]
              tunnel: w414 -> [_ w420]
              tunnel: [_ w419] -> w412
              frame False {
              }
              frame True {
                n165 = call-poly <vilib>:"Delacor_lib_QMH_Enqueue Message (poly).vi"("Message Data"=w420, "Message"="Validate connection", "Message Queue in"=w422) -> ("error out"=w419:errorcluster)  [unwired: 7 in, 1 out]
              }
            }
          }
          event User Event {
            # "Another Module called the \"Start continous acquisition\" API Method."
            n166 = event-data() -> ("Module ID"=w428:i32, "Task list"=w427:T4, "Timeout"=w426:i32, "Acq type"=w425:enum16{"Single", "Multiple"}, "N samples"=w424:i32)  [unwired: 1 in]
            n167 = Bundle(cluster=T23 {"Module ID"=-1, "Task list"=enum."All", "Timeout"=0, "Acq type"=enum."Single", "N samples"=0, "Data in"=variant} ("Start continous acquisition Argument"), "Module ID"=w428, "Task list"=w427, "Timeout"=w426, "Acq type"=w425, "N samples"=w424) -> (w429:T23)  [unwired: 1 in]
            n168 = call "Addressed to This Module.vi"("Module ID from Argument"=w428, "Module Admin"=w431) -> ("Addressed to this instance?"=w432:bool)  [unwired: 8 in, 1 out]
            n169 = case shown="True" w432 {
              tunnel: w433 -> [_ w437]
              tunnel: w429 -> [_ w435]
              tunnel: [_ w434] -> w423
              frame False {
              }
              frame True {
                n170 = call-poly <vilib>:"Delacor_lib_QMH_Enqueue Message (poly).vi"("Message Data"=w435, "Message"="Start continous acquisition", "Message Queue in"=w437) -> ("error out"=w434:errorcluster)  [unwired: 7 in, 1 out]
              }
            }
          }
          event User Event {
            # "Another Module called the \"Stop continuous acquisition\" API Method."
            n171 = event-data() -> ("Module ID"=w440:i32, "Boolean"=w439:bool)  [unwired: 1 in]
            n172 = Bundle(cluster=T24 {"Module ID"=-1, "Boolean"=FALSE} ("Stop continuous acquisition Argument"), "Module ID"=w440, "Boolean"=w439) -> (w441:T24)
            n173 = call "Addressed to This Module.vi"("Module ID from Argument"=w440, "Module Admin"=w443) -> ("Addressed to this instance?"=w444:bool)  [unwired: 8 in, 1 out]
            n174 = case shown="True" w444 {
              tunnel: w445 -> [_ w449]
              tunnel: w441 -> [_ w447]
              tunnel: [_ w446] -> w438
              frame False {
              }
              frame True {
                n175 = call-poly <vilib>:"Delacor_lib_QMH_Enqueue Message (poly).vi"("Message Data"=w447, "Message"="Stop continuous acquisition", "Message Queue in"=w449) -> ("error out"=w446:errorcluster)  [unwired: 7 in, 1 out]
              }
            }
          }
        }
        n176 = call-dynamic "Delacor_lib_QMH_Error Handler - Event Handling Loop.vi"("error in"=w154, "Message Queue in"=w148) -> ("dup error in"=w153:errorcluster)  [unwired: 8 in, 1 out]
      }
      n177 = while {
        tunnel: w37 -> [w454]
        shift-right: [w458] -> _
        shift-left: T5 {"Status"="", "DO task"="", "DI task"="", "AO task"="", "AI task"="", "Device name"=""} ("Data Cluster") -> [w459]
        tunnel: w41 -> [w462]
        tunnel: [w460] -> w43
        tunnel: w36 -> [w452]
        tunnel: [w451] -> w35
        tunnel: w28 -> [w450]
        stop <- w457 stop-if-true
        # "Message Handling Loop"
        n178 = call-dynamic "Delacor_lib_QMH_Dequeue Message.vi"("error in"=w462, "Message Queue in"=w454) -> ("error out"=w461:errorcluster, "Message Data"=w455:variant, "Message"=w456:string, "Message Queue out"=w453:refnum<class "Delacor_lib_QMH_Message Queue.lvclass">)  [unwired: 6 in]
        n179 = case "DQMH_MESSAGE_CASES" shown="\"Stop task\"" w456 {
          selector: w456 -> [_ _ _ _ _ _ _ _ _ _ _ _ _ _ _ _ _ w861 _ _ _]
          tunnel: w453 -> [_ _ _ _ _ _ _ _ _ _ _ _ _ _ _ w818 w852 _ _ _ _]
          tunnel: w461 -> [w494 w512 w529 w545 w581 w648 w668 w685 w702 w713 w735 w761 w780 w803 w816 w827 w857 w863 w890 w920 w939]
          tunnel: [w492 w505 w515 w533 w574 w634 w654 w679 w693 w704 w726 w752 w774 w794 w816 w823 w855 w864 w881 w910 w933] -> w463
          tunnel: w459 -> [w485 w508 w520 w540 w577 w629 w663 w680 w697 w707 w724 w750 w773 w792 w815 w822 w842 w862 w880 w906 w938]
          tunnel: [w484 w507 w520 w540 w577 w628 w663 w680 w697 w707 w724 w750 w773 w792 w815 w822 w842 w862 w880 w906 w938] -> w458
          tunnel: [_ _ _ _ _ _ _ _ _ _ _ _ _ _ _ _ w851 _ _ _ _] -> w457
          tunnel: w455 -> [_ w511 w527 w543 w580 w646 w667 w684 w701 w711 w733 w759 w779 w801 _ w821 w849 _ w888 w919 w937]
          tunnel: w452 -> [w479 _ _ _ _ _ _ _ _ _ _ _ _ _ _ w820 w845 w859 _ _ _]
          tunnel: [_ _ _ _ _ _ _ _ _ _ _ _ _ _ _ _ w847 _ _ _ _] -> w451
          tunnel: w450 -> [_ _ _ _ _ _ _ _ _ _ _ _ _ _ _ _ _ _ _ w909 w932]
          frame "Initialize" {
            w476 = "Initial Message" ("Initial Message")
            # "#TODO:  create a task for each kind of channel."
            # "Initialize - Any operation that needs to be done before the module can receive messages. Synchronize Caller Events.vi will inform Start Module.vi that the module has launched and is ready to receive messages. Module Did Init.vi will broadcast that the module initialized."
            n180 = call "Synchronize Caller Events.vi"("error in (no error)"=w494, "Module Admin"=w479) -> ("error out"=w493:errorcluster, "Module Admin out"=w478:refnum<class "Delacor_lib_QMH_Cloneable Module Admin.lvclass">)  [unwired: 8 in]
            n181 = call <vilib>:"Create NI GUID.vi"() -> ("NI GUID"=w475:string)
            n182 = property class="Mod Admin"(reference=w478) -> ("Accessors:Module ID"=w481:i32, "Accessors:External Launch"=w480:bool)  [unwired: 1 in, 2 out]
            n183 = for {
              tunnel: w475 -> [w500]
              tunnel: " %s" ("format string") -> [w499]
              tunnel: string[] ["DO task", "DI task", "AO task", "AI task"] ("new task name") -> [w498] mode=indexing
              tunnel: [w497] -> w468 mode=indexing
              n184 = Format Into String(format string=w499, initial string=w498, w500) -> (resulting string=w497:string)  [unwired: 1 in, 1 out]
            }
            n185 = call "Module Name--constant.vi"("Module ID"=w481) -> ("Module Name"=w489:string)  [unwired: 10 in]
            n186 = Index Array(array=w468) -> (element #1=w464:string, element #2=w465:string, element #3=w466:string, element #4=w467:string)  [unwired: 4 in]
            n187 = property class="VI"("Front Panel.Title"=w489) -> (reference out=w491:refnum<vi>, error out=w496:errorcluster)  [unwired: 2 in]
            n188 = Select(t=T26."Hidden" ("State"), s=w480, f=T26."Standard" ("State")) -> (s? t:f=w486:T26)
            n189 = call <vilib>:"DAQmx Create Task.vi"("new task name"=w464) -> ("task out"=w474:refnum<k21>)  [unwired: 13 in, 1 out]
            n190 = call <vilib>:"DAQmx Create Task.vi"("new task name"=w465) -> ("task out"=w473:refnum<k21>)  [unwired: 13 in, 1 out]
            n191 = call <vilib>:"DAQmx Create Task.vi"("new task name"=w466) -> ("task out"=w472:refnum<k21>)  [unwired: 13 in, 1 out]
            n192 = call <vilib>:"DAQmx Create Task.vi"("new task name"=w467) -> ("task out"=w471:refnum<k21>)  [unwired: 13 in, 1 out]
            n193 = invoke class="VI" method="FP.Open"(reference=w491, error in=w496, "State"=w486) -> (reference out=w490:refnum<vi>, error out=w495:errorcluster)  [unwired: 2 in, 3 out]
            n194 = Bundle By Name(cluster=w485, "DO task"=w474, "DI task"=w473, "AO task"=w472, "AI task"=w471, "Status"=w476) -> (w484:T5)
            n195 = call "Module Name--constant.vi"("Module ID"=w481) -> ("Module Name"=w482:string)  [unwired: 10 in]
            n196 = invoke class="VI" method="FP.Center"(reference=w490, error in=w495) -> ()  [unwired: 1 in, 3 out]
            n197 = property on="Pane" class="Pane"("Origin"=T25 {"Horizontal"=0, "Vertical"=0}) -> ()  [unwired: 2 in, 2 out]
            n198 = call "Module Did Init.vi"("error in (no error)"=w493, "Initialized?"=TRUE, "Origin"=w482, "Module ID"=w481) -> ("error out"=w492:errorcluster)  [unwired: 7 in]
            "Status" <- w476
          }
          frame "Set device ID" {
            # "Set the device identifier to be managed internally by the module."
            n199 = Variant To Data(error in=w512, type=T8 {"Module ID"=-1, "Device ID"=""} ("Set device ID Argument"), Variant=w511) -> (data=w509:T8, error out=w506:errorcluster)
            n200 = Unbundle By Name(w509) -> ("Device ID"=w501:tag, "Module ID"=w504:i32)
            n201 = Bundle By Name(cluster=w508, "Device name"=w501) -> (w507:T5)
            n202 = Format Into String(format string="Device ID set to %s.", w501) -> (resulting string=w502:string)  [unwired: 2 in, 1 out]
            n203 = call "Status Updated.vi"("error in (no error)"=w506, "Status"=w502, "Module ID"=w504) -> ("error out"=w505:errorcluster)  [unwired: 8 in]
          }
          frame "Get channel list" {
            # "Request to read all available channels from the specified device."
            n204 = Variant To Data(error in=w529, type=T9 {"Module ID"=-1, "Wait Notifier"=refnum, "wait for reply"=FALSE} ("Get channel list Argument"), Variant=w527) -> (data=w525:T9, error out=w528:errorcluster)
            n205 = Unbundle By Name(w520) -> ("Device name"=w519:tag)
            n206 = Unbundle By Name(w525) -> ("Wait Notifier"=w524:refnum<notifier>, "wait for reply"=w523:bool, "Module ID"=w514:i32)
            n207 = call "Get Channels.vi"("Active device"=w519) -> ("error out"=w518:errorcluster, "Available channels"=w517:i32)  [unwired: 9 in]
            n208 = Bundle By Name(cluster=T27 {"Available channels"=0, "error"={"status"=FALSE, "code"=0, "source"=""}} ("Get channel list (Reply Payload)"), "Available channels"=w517, "error"=w518) -> (w522:T27)
            n209 = Merge Errors(w528, w518) -> (w516:errorcluster)
            n210 = case shown="True" w523 {
              tunnel: w524 -> [_ w531]
              tunnel: w522 -> [_ w530]
              frame False {
              }
              frame True {
                n211 = Send Notification(notification=w530, notifier=w531) -> ()  [unwired: 1 in, 2 out]
              }
            }
            n212 = call "Status Updated.vi"("error in (no error)"=w516, "Status"="Channel list updated.", "Module ID"=w514) -> ("error out"=w515:errorcluster)  [unwired: 8 in]
          }
          frame "Start task" {
            # "Request to start all existing channels for the local task."
            n213 = Unbundle By Name(w540) -> ("DO task"=w539:refnum<k21>, "DI task"=w538:refnum<k21>, "AO task"=w537:refnum<k21>, "AI task"=w536:refnum<k21>)
            n214 = Variant To Data(error in=w545, type=T11 {"Module ID"=-1, "Boolean"=FALSE} ("Start task Argument"), Variant=w543) -> (data=w541:T11, error out=w544:errorcluster)
            n215 = Unbundle By Name(w541) -> ("Module ID"=w532:i32)
            n216 = Build Array(w539, w538, w537, w536) -> (w534:refnum<k21>[])
            n217 = for {
              tunnel: [w548] -> w535
              tunnel: w534 -> [w550] mode=indexing
              tunnel: w532 -> [w546]
              n218 = call <vilib>:"DAQmx Start Task.vi"("task/channels in"=w550) -> ("task out"=w547:refnum<k21>, "error out"=w549:errorcluster)  [unwired: 13 in]
              n219 = case shown="No Error" w549 {
                selector: w549 -> [w555 w558 w561]
                tunnel: [w556 w559 w565] -> w548
                tunnel: w547 -> [w553 _ _]
                tunnel: w546 -> [w551 _ w563]
                frame No Error {
                  n220 = Format Into String(format string="Task %s started successfuly." ("Status"), w553) -> (resulting string=w552:string)  [unwired: 2 in, 1 out]
                  n221 = call "Status Updated.vi"("error in (no error)"=w555, "Status"=w552, "Module ID"=w551) -> ("error out"=w556:errorcluster)  [unwired: 8 in]
                }
                frame Error {
                  # "Task has no channels"
                  n222 = call <vilib>:"Clear Errors.vi"("error in (no error)"=w558, "specific error code to clear (0: all)"=-200478) -> ("error out"=w559:errorcluster)  [unwired: 4 in, 1 out]
                }
                frame Default {
                  # "Unknown error"
                  n223 = call <vilib>:"Clear Errors.vi"("error in (no error)"=w561) -> ("error out"=w566:errorcluster)  [unwired: 5 in, 1 out]
                  n224 = Unbundle By Name(w561) -> ("code"=w560:i32)
                  n225 = Format Into String(format string="Unknown error while starting task. Error code: %d." ("Status"), w560) -> (resulting string=w564:string)  [unwired: 2 in, 1 out]
                  n226 = call "Status Updated.vi"("error in (no error)"=w566, "Status"=w564, "Module ID"=w563) -> ("error out"=w565:errorcluster)  [unwired: 8 in]
                }
              }
            }
            n227 = Merge Errors(w544, w535) -> (w533:errorcluster)
          }
          frame "Stop task" {
            # "Request to stop all channels within the local task."
            n228 = Variant To Data(error in=w581, type=T12 {"Module ID"=-1, "Task list"=enum."All"} ("Stop task Argument"), Variant=w580) -> (data=w578:T12, error out=w576:errorcluster)
            n229 = Unbundle By Name(w577) -> ("DO task"=w573:refnum<k21>, "DI task"=w572:refnum<k21>, "AO task"=w571:refnum<k21>, "AI task"=w570:refnum<k21>)
            n230 = Unbundle By Name(w578) -> ("Task list"=w569:T4, "Module ID"=w567:i32)
            n231 = Build Array(w573, w572, w571, w570) -> (w568:refnum<k21>[])
            n232 = case shown="\"All\", Default" w569 {
              tunnel: [w583 w596 w602 w609 w619] -> w575
              tunnel: w568 -> [w586 w597 w599 w608 w617]
              tunnel: w567 -> [w584 w594 w601 w610 w618]
              frame "All", Default {
                n233 = for {
                  tunnel: w586 -> [w589] mode=indexing
                  shift-right: [w588] -> w582
                  shift-left: _ -> [w587]
                  n234 = call <vilib>:"DAQmx Stop Task.vi"("task/channels in"=w589, "error in"=w587) -> ("error out"=w588:errorcluster)  [unwired: 12 in, 1 out]
                }
                n235 = call "Status Updated.vi"("error in (no error)"=w582, "Status"="All tasks stopped. Standing by.", "Module ID"=w584) -> ("error out"=w583:errorcluster)  [unwired: 8 in]
              }
              frame "DO task" {
                n236 = Index Array(array=w597) -> (element=w593:refnum<k21>)  [unwired: 1 in]
                n237 = call <vilib>:"DAQmx Stop Task.vi"("task/channels in"=w593) -> ("task out"=w590:refnum<k21>, "error out"=w595:errorcluster)  [unwired: 13 in]
                n238 = Format Into String(format string="Task %s stopped. Standing by." ("Status"), w590) -> (resulting string=w591:string)  [unwired: 2 in, 1 out]
                n239 = call "Status Updated.vi"("error in (no error)"=w595, "Status"=w591, "Module ID"=w594) -> ("error out"=w596:errorcluster)  [unwired: 8 in]
              }
              frame "DI task" {
                n240 = Index Array(array=w599, index=1) -> (element=w600:refnum<k21>)
                n241 = call <vilib>:"DAQmx Stop Task.vi"("task/channels in"=w600) -> ("task out"=w603:refnum<k21>, "error out"=w606:errorcluster)  [unwired: 13 in]
                n242 = Format Into String(format string="Task %s stopped. Standing by." ("Status"), w603) -> (resulting string=w604:string)  [unwired: 2 in, 1 out]
                n243 = call "Status Updated.vi"("error in (no error)"=w606, "Status"=w604, "Module ID"=w601) -> ("error out"=w602:errorcluster)  [unwired: 8 in]
              }
              frame "AO task" {
                n244 = Index Array(array=w608, index=2) -> (element=w614:refnum<k21>)
                n245 = call <vilib>:"DAQmx Stop Task.vi"("task/channels in"=w614) -> ("task out"=w611:refnum<k21>, "error out"=w615:errorcluster)  [unwired: 13 in]
                n246 = Format Into String(format string="Task %s stopped. Standing by." ("Status"), w611) -> (resulting string=w612:string)  [unwired: 2 in, 1 out]
                n247 = call "Status Updated.vi"("error in (no error)"=w615, "Status"=w612, "Module ID"=w610) -> ("error out"=w609:errorcluster)  [unwired: 8 in]
              }
              frame "AI task" {
                n248 = Index Array(array=w617, index=3) -> (element=w622:refnum<k21>)
                n249 = call <vilib>:"DAQmx Stop Task.vi"("task/channels in"=w622) -> ("task out"=w624:refnum<k21>, "error out"=w621:errorcluster)  [unwired: 13 in]
                n250 = Format Into String(format string="Task %s stopped. Standing by." ("Status"), w624) -> (resulting string=w623:string)  [unwired: 2 in, 1 out]
                n251 = call "Status Updated.vi"("error in (no error)"=w621, "Status"=w623, "Module ID"=w618) -> ("error out"=w619:errorcluster)  [unwired: 8 in]
              }
            }
            n252 = Merge Errors(w576, w575) -> (w574:errorcluster)
          }
          frame "Create DO channel" {
            # "Request to create a digital output task from the selected lines."
            n253 = Variant To Data(error in=w648, type=T10 {"Module ID"=-1, "lines"="", "Wait Notifier"=refnum, "wait for reply"=FALSE, "Channel name"=""} ("Create DO task Argument"), Variant=w646) -> (data=w644:T10, error out=w647:errorcluster)
            n254 = Unbundle By Name(w629) -> ("DO task"=w627:refnum<k21>, "Device name"=w637:tag)
            n255 = Unbundle By Name(w644) -> ("Wait Notifier"=w643:refnum<notifier>, "wait for reply"=w642:bool, "lines"=w636:tag, "Channel name"=w625:string, "Module ID"=w633:i32)
            n256 = Format Into String(format string="%s/%s", w637, w636) -> (resulting string=w631:string)  [unwired: 2 in, 1 out]
            n257 = call-poly <vilib>:"DAQmx Create Virtual Channel.vi"("task in"=w627, "lines"=w631, "name to assign"=w625) -> ("task out"=w626:refnum<k21>, "error out"=w639:errorcluster)  [unwired: 11 in]
            n258 = Bundle By Name(cluster=w629, "DO task"=w626) -> (w628:T5)
            n259 = Merge Errors(w647, w639) -> (w635:errorcluster)
            n260 = Format Into String(format string="Channel %s created. Standing by.", w625) -> (resulting string=w630:string)  [unwired: 2 in, 1 out]
            n261 = Bundle By Name(cluster=T28 {"task out"="", "error"={"status"=FALSE, "code"=0, "source"=""}} ("Create DO task (Reply Payload)"), "task out"=w626, "error"=w639) -> (w641:T28)
            n262 = case shown="True" w642 {
              tunnel: w643 -> [_ w650]
              tunnel: w641 -> [_ w649]
              frame False {
              }
              frame True {
                n263 = Send Notification(notification=w649, notifier=w650) -> ()  [unwired: 1 in, 2 out]
              }
            }
            n264 = call "Status Updated.vi"("error in (no error)"=w635, "Status"=w630, "Module ID"=w633) -> ("error out"=w634:errorcluster)  [unwired: 8 in]
          }
          frame "Create DI channel" {
            # "Request to create a digital input channel(s)."
            n265 = Variant To Data(error in=w668, type=T14 {"Module ID"=-1, "Physical channel"="", "Channel name"=""} ("Create DI channel Argument"), Variant=w667) -> (data=w665:T14, error out=w656:errorcluster)
            n266 = Unbundle By Name(w663) -> ("DI task"=w661:refnum<k21>, "Device name"=w662:tag)
            n267 = Unbundle By Name(w665) -> ("Physical channel"=w660:string, "Channel name"=w659:string, "Module ID"=w651:i32)
            n268 = Format Into String(format string="%s/%s", w662, w660) -> (resulting string=w653:string)  [unwired: 2 in, 1 out]
            n269 = call-poly <vilib>:"DAQmx Create Virtual Channel.vi"("task in"=w661, "lines"=w653, "name to assign"=w659) -> ("error out"=w657:errorcluster)  [unwired: 11 in, 1 out]
            n270 = Merge Errors(w656, w657) -> (w655:errorcluster)
            n271 = Format Into String(format string="Channel %s created. Standing by.", w653) -> (resulting string=w652:string)  [unwired: 2 in, 1 out]
            n272 = call "Status Updated.vi"("error in (no error)"=w655, "Status"=w652, "Module ID"=w651) -> ("error out"=w654:errorcluster)  [unwired: 8 in]
          }
          frame "Create AI channel" {
            # "Request to create an analog input channel in the selected channel."
            n273 = Variant To Data(error in=w685, type=T17 {"Module ID"=-1, "Physical channel"="", "Channel name"="", "Config params"={"input terminal configuration"=-1, "minimum value"=-5.0, "maximum value"=5.0}} ("Create AI channel Argument"), Variant=w684) -> (data=w682:T17, error out=w681:errorcluster)
            n274 = Unbundle By Name(w682) -> ("Config params"=w677:T33, "Physical channel"=w671:string, "Channel name"=w672:string)
            n275 = Unbundle By Name(w680) -> ("AI task"=w670:refnum<k21>, "Device name"=w669:tag)
            n276 = Unbundle By Name(w677) -> ("input terminal configuration"=w676:i32, "minimum value"=w675:dbl, "maximum value"=w674:dbl)
            n277 = Format Into String(format string="%s/%s", w669, w671) -> (resulting string=w673:string)  [unwired: 2 in, 1 out]
            n278 = call-poly <vilib>:"DAQmx Create Virtual Channel.vi"("task in"=w670, "maximum value"=w674, "minimum value"=w675, "input terminal configuration"=w676, "physical channels"=w673, "name to assign"=w672, "error in"=w681) -> ("error out"=w679:errorcluster)  [unwired: 7 in, 1 out]
          }
          frame "Create AO channel" {
            # "Request to create single or multiple analog output channel (s)."
            n279 = Variant To Data(error in=w702, type=T19 {"Module ID"=-1, "Physical channel"="", "Channel name"="", "Config params"={"Terminal configuration"=-1, "min value"=-5.0, "max value"=5.0}} ("Create AO channel Argument"), Variant=w701) -> (data=w699:T19, error out=w694:errorcluster)
            n280 = Unbundle By Name(w699) -> ("Config params"=w689:T20, "Physical channel"=w695:string, "Channel name"=w690:string)
            n281 = Unbundle By Name(w697) -> ("AO task"=w692:refnum<k21>, "Device name"=w696:tag)
            n282 = Unbundle By Name(w689) -> ("Terminal configuration"=w688:i32, "min value"=w687:dbl, "max value"=w686:dbl)
            n283 = Format Into String(format string="%s/%s", w696, w695) -> (resulting string=w691:string)  [unwired: 2 in, 1 out]
            n284 = call-poly <vilib>:"DAQmx Create Virtual Channel.vi"("task in"=w692, "maximum value"=w686, "minimum value"=w687, "output terminal configuration"=w688, "physical channels"=w691, "name to assign"=w690, "error in"=w694) -> ("error out"=w693:errorcluster)  [unwired: 7 in, 1 out]
          }
          frame "Write DO" {
            # "Request to write to a single or multiple digital output channels."
            n285 = Variant To Data(error in=w713, type=T13 {"Module ID"=-1, "Samples"=enum."Single", "Data"=[]} ("Write DO Argument"), Variant=w711) -> (data=w709:T13, error out=w712:errorcluster)
            n286 = Unbundle By Name(w707) -> ("DO task"=w706:refnum<k21>)
            n287 = Unbundle By Name(w709) -> ("Data"=w705:bool[], "Samples"=w708:enum16{"Single", "Multiple"})
            n288 = case shown="\"Single\", Default" w708 {
              tunnel: w706 -> [w716 w720]
              tunnel: w705 -> [w715 w718]
              tunnel: [w717 w719] -> w703
              frame "Single", Default {
                n289 = Index Array(array=w715) -> (element=w714:bool)  [unwired: 1 in]
                n290 = call-poly <vilib>:"DAQmx Write.vi"("task/channels in"=w716, "data"=w714) -> ("error out"=w717:errorcluster)  [unwired: 11 in, 2 out]
              }
              frame "Multiple" {
                n291 = call-poly <vilib>:"DAQmx Write.vi"("task/channels in"=w720, "data"=w718) -> ("error out"=w719:errorcluster)  [unwired: 11 in, 2 out]
              }
            }
            n292 = Merge Errors(w712, w703) -> (w704:errorcluster)
          }
          frame "Read DI" {
            # "Request to read one or multiple digital inputs."
            n293 = Variant To Data(error in=w735, type=T15 {"Module ID"=-1, "Samples"=enum."Single", "Wait Notifier"=refnum, "wait for reply"=FALSE} ("Read DI Argument"), Variant=w733) -> (data=w731:T15, error out=w734:errorcluster)
            n294 = Unbundle By Name(w731) -> ("Wait Notifier"=w730:refnum<notifier>, "wait for reply"=w729:bool, "Samples"=w725:enum16{"Single", "Multiple"})
            n295 = Unbundle By Name(w724) -> ("DI task"=w723:refnum<k21>)
            n296 = case shown="\"Multiple\"" w725 {
              tunnel: w723 -> [w739 w744]
              tunnel: [w737 w742] -> w722
              tunnel: [w736 w743] -> w721
              frame "Single", Default {
                n297 = call-poly <vilib>:"DAQmx Read.vi"("task/channels in"=w739) -> ("data"=w738:bool, "error out"=w736:errorcluster)  [unwired: 12 in, 1 out]
                n298 = Build Array(w738) -> (w737:bool[])
              }
              frame "Multiple" {
                n299 = call-poly <vilib>:"DAQmx Read.vi"("task/channels in"=w744) -> ("data"=w741:u8[], "error out"=w743:errorcluster)  [unwired: 12 in, 1 out]
                n300 = Index Array(array=w741) -> (element=w740:u8)  [unwired: 1 in]
                n301 = Number To Boolean Array(number=w740) -> (Boolean array=w742:bool[])
              }
            }
            n302 = Merge Errors(w734, w721) -> (w726:errorcluster)
            n303 = Bundle By Name(cluster=T29 {"Data"=[], "error"={"status"=FALSE, "code"=0, "source"=""}} ("Read DI (Reply Payload)"), "Data"=w722, "error"=w721) -> (w728:T29)
            n304 = case shown="True" w729 {
              tunnel: w730 -> [_ w746]
              tunnel: w728 -> [_ w745]
              frame False {
              }
              frame True {
                n305 = Send Notification(notification=w745, notifier=w746) -> ()  [unwired: 1 in, 2 out]
              }
            }
          }
          frame "Read AI" {
            # "Request to read single or multiple analog inputs."
            n306 = Variant To Data(error in=w761, type=T18 {"Module ID"=-1, "Samples"=enum."Single", "Wait Notifier"=refnum, "wait for reply"=FALSE} ("Read AI Argument"), Variant=w759) -> (data=w757:T18, error out=w760:errorcluster)
            n307 = Unbundle By Name(w757) -> ("Wait Notifier"=w756:refnum<notifier>, "wait for reply"=w755:bool, "Samples"=w751:enum16{"Single", "Multiple"})
            n308 = Unbundle By Name(w750) -> ("AI task"=w749:refnum<k21>)
            n309 = case shown="\"Single\"" w751 {
              tunnel: w749 -> [w764 w768]
              tunnel: [w763 w765] -> w748
              tunnel: [w762 w767] -> w747
              frame "Multiple", Default {
                n310 = call-poly <vilib>:"DAQmx Read.vi"("task/channels in"=w764) -> ("data"=w763:dbl[], "error out"=w762:errorcluster)  [unwired: 12 in, 1 out]
              }
              frame "Single" {
                n311 = call-poly <vilib>:"DAQmx Read.vi"("task/channels in"=w768) -> ("data"=w766:dbl, "error out"=w767:errorcluster)  [unwired: 12 in, 1 out]
                n312 = Build Array(w766) -> (w765:dbl[])
              }
            }
            n313 = Bundle By Name(cluster=T30 {"Data"=[], "error"={"status"=FALSE, "code"=0, "source"=""}} ("Read AI (Reply Payload)"), "Data"=w748, "error"=w747) -> (w754:T30)
            n314 = Merge Errors(w760, w747) -> (w752:errorcluster)
            n315 = case shown="True" w755 {
              tunnel: w756 -> [_ w770]
              tunnel: w754 -> [_ w769]
              frame False {
              }
              frame True {
                n316 = Send Notification(notification=w769, notifier=w770) -> ()  [unwired: 1 in, 2 out]
              }
            }
          }
          frame "Write AO" {
            # "Request to write a value to a single or multiple channel (s)"
            n317 = Variant To Data(error in=w780, type=T21 {"Module ID"=-1, "Value(s)"=[], "Samples"=enum."Single"} ("Write AO Argument"), Variant=w779) -> (data=w777:T21, error out=w775:errorcluster)
            n318 = Unbundle By Name(w773) -> ("AO task"=w772:refnum<k21>)
            n319 = Unbundle By Name(w777) -> ("Samples"=w776:enum16{"Single", "Multiple"}, "Value(s)"=w771:dbl[])
            n320 = case shown="\"Multiple\", Default" w776 {
              tunnel: w775 -> [w785 w789]
              tunnel: [w784 w788] -> w774
              tunnel: w772 -> [w783 w787]
              tunnel: w771 -> [w782 w786]
              frame "Multiple", Default {
                n321 = Index Array(array=w782) -> (element=w781:dbl)  [unwired: 1 in]
                n322 = call-poly <vilib>:"DAQmx Write.vi"("task/channels in"=w783, "data"=w781, "error in"=w785) -> ("error out"=w784:errorcluster)  [unwired: 10 in, 2 out]
              }
              frame "Single" {
                n323 = call-poly <vilib>:"DAQmx Write.vi"("task/channels in"=w787, "data"=w786, "error in"=w789) -> ("error out"=w788:errorcluster)  [unwired: 10 in, 2 out]
              }
            }
          }
          frame "Get task ref" {
            # "Request to get a reference to a given task."
            n324 = Variant To Data(error in=w803, type=T16 {"Module ID"=-1, "Task list"=enum."All", "Wait Notifier"=refnum, "wait for reply"=FALSE} ("Get task ref Argument"), Variant=w801) -> (data=w799:T16, error out=w802:errorcluster)
            n325 = Unbundle By Name(w799) -> ("Task list"=w793:T4, "Wait Notifier"=w798:refnum<notifier>, "wait for reply"=w797:bool)
            n326 = case shown="\"DO task\"" w793 {
              tunnel: w792 -> [_ w806 w808 w810 w812]
              tunnel: [_ w805 w807 w809 w811] -> w791
              tunnel: [errorcluster {"status"=FALSE, "code"=0, "source"=""} ("error in (no error)") _ _ _ _] -> w790
              frame "All", Default {
              }
              frame "DO task" {
                n327 = Unbundle By Name(w806) -> ("DO task"=w805:refnum<k21>)
              }
              frame "DI task" {
                n328 = Unbundle By Name(w808) -> ("DI task"=w807:refnum<k21>)
              }
              frame "AO task" {
                n329 = Unbundle By Name(w810) -> ("AO task"=w809:refnum<k21>)
              }
              frame "AI task" {
                n330 = Unbundle By Name(w812) -> ("AI task"=w811:refnum<k21>)
              }
            }
            n331 = Bundle By Name(cluster=T31 {"DAQmx Task"="", "error"={"status"=FALSE, "code"=0, "source"=""}} ("Get task ref (Reply Payload)"), "DAQmx Task"=w791, "error"=w790) -> (w796:T31)
            n332 = Merge Errors(w802, w790) -> (w794:errorcluster)
            n333 = case shown="True" w797 {
              tunnel: w798 -> [_ w814]
              tunnel: w796 -> [_ w813]
              frame False {
              }
              frame True {
                n334 = Send Notification(notification=w813, notifier=w814) -> ()  [unwired: 1 in, 2 out]
              }
            }
          }
          frame "---Exit and Error Handling---" {
            # "Separator - the following cases handle errors and exit messages."
          }
          frame "Error" {
            # "#CodeRecommended - If you ever change the name of this \"Error\" message, you'll need to update the name in the Check Loop Error.vi as well."
            # "#CodeRecommended - If the module is running in standalone mode (External Launch = FALSE), this code will pop up an error dialog and call the 'Exit' message if an error occurs. Add more fine-grained error handling here."
            # "Error - Check the error message data and respond accordingly. This message is sent by the \"Error Handler\" VIs at the end of each loop in this application."
            n335 = property class="Mod Admin"(reference=w820) -> ("Accessors:External Launch"=w819:bool, "Accessors:Module ID"=w817:i32)  [unwired: 1 in, 2 out]
            n336 = Variant To Data(error in=w827, type=errorcluster {"status"=FALSE, "code"=0, "source"=""} ("error constant"), Variant=w821) -> (data=w828:errorcluster, error out=w825:errorcluster)
            n337 = call "Error Reported.vi"("Error"=w828, "Module ID"=w817) -> ()  [unwired: 9 in, 1 out]
            n338 = case shown="False" w819 {
              tunnel: [w833 _] -> w824
              tunnel: w818 -> [w831 _]
              tunnel: w828 -> [w832 _]
              frame False {
                # "If the module is running standalone, then pop up an error dialog and call the \"Exit\" message."
                n339 = call <vilib>:"Simple Error Handler.vi"("error in (no error)"=w832) -> ()  [unwired: 4 in, 5 out]
                n340 = call-poly <vilib>:"Delacor_lib_QMH_Enqueue Message (poly).vi"("Priority Message? (F)"=TRUE, "Message"="Exit", "Message Queue in"=w831) -> ("error out"=w833:errorcluster)  [unwired: 7 in, 1 out]
              }
              frame True {
                # "If the module was launched externally, calling the Error Reported broadcast VI is the only action performed by the \"Error\" message. The module's caller can then process the error appropriately."
              }
            }
            n341 = Merge Errors(w825, w824) -> (w823:errorcluster)
            n342 = local write "error out"(w823) -> ()
          }
          frame "Exit" {
            w850 = 91  # 91: not all Exit messages will have an argument
            w851 = TRUE  # Stop the VI
            # "Release the message queue reference"
            # "Exit - Exit the application."
            n343 = Variant To Data(error in=w857, type=T7 {"Module ID"=-1, "Origin"="", "Exit via Stop Module Req?"=FALSE, "Wait for Module to stop?"=FALSE} ("Stop Argument"), Variant=w849) -> (data=w846:T7, error out=w853:errorcluster)
            n344 = call <vilib>:"Clear Errors.vi"("error in (no error)"=w853, "specific error code to clear (0: all)"=w850) -> ("error out"=w856:errorcluster)  [unwired: 4 in, 1 out]
            n345 = Unbundle By Name(w842) -> ("DO task"=w834:refnum<k21>, "DI task"=w835:refnum<k21>, "AO task"=w836:refnum<k21>, "AI task"=w841:refnum<k21>)
            n346 = call-dynamic "Delacor_lib_QMH_Release Message Queue.vi"("error in"=w856, "Message Queue"=w852) -> ("error out"=w843:errorcluster)  [unwired: 9 in]
            n347 = control-ref of="This VI"() -> (w844:refnum<vi>)
            n348 = call <vilib>:"DAQmx Clear Task.vi"("task in"=w841, "error in"=w843) -> ("error out"=w840:errorcluster)  [unwired: 13 in]
            n349 = call "Handle Exit.vi"("Stop Argument"=w846, "Module Admin in"=w845, "VI reference"=w844) -> ("error out"=w854:errorcluster, "Wait for Stop?"=w847:bool)  [unwired: 7 in]
            n350 = call <vilib>:"DAQmx Clear Task.vi"("task in"=w836, "error in"=w840) -> ("error out"=w839:errorcluster)  [unwired: 13 in]
            n351 = call <vilib>:"DAQmx Clear Task.vi"("task in"=w835, "error in"=w839) -> ("error out"=w838:errorcluster)  [unwired: 13 in]
            n352 = call <vilib>:"DAQmx Clear Task.vi"("task in"=w834, "error in"=w838) -> ("error out"=w837:errorcluster)  [unwired: 13 in]
            n353 = Merge Errors(w837, w854) -> (w855:errorcluster)
          }
          frame Default {
            # "'Default' case only runs if there is a message that isn't defined in any of the other cases.  Output a programming error."
            n354 = property class="Mod Admin"(reference=w859) -> ("Accessors:Module ID"=w858:i32)  [unwired: 1 in, 2 out]
            n355 = call "Module Name--constant.vi"("Module ID"=w858) -> ("Module Name"=w860:string)  [unwired: 10 in]
            n356 = xnode "Error Ring"("parameter 0"=w861, "parameter 1"=w860) -> ("error out"=w865:errorcluster)
            n357 = Merge Errors(w863, w865) -> (w864:errorcluster)
          }
          frame "Validate connection" {
            # "Request to validate correct connection to device. Call after the Set device ID event."
            n358 = property class="DAQmx System"() -> (error out=w879:errorcluster, "DevNames"=w876:tag[])  [unwired: 2 in, 1 out]
            n359 = Unbundle By Name(w880) -> ("Device name"=w875:tag)
            n360 = Variant To Data(error in=w890, type=T22 {"Module ID"=-1, "Wait Notifier"=refnum, "wait for reply"=FALSE} ("Validate connection Argument"), Variant=w888) -> (data=w886:T22, error out=w889:errorcluster)
            n361 = Unbundle By Name(w886) -> ("Module ID"=w877:i32, "Wait Notifier"=w885:refnum<notifier>, "wait for reply"=w884:bool)
            n362 = for {
              tunnel: w876 -> [w900] mode=indexing
              tunnel: w875 -> [w901]
              tunnel: [w899] -> w874
              stop <- w899 stop-if-true
              n363 = Equal?(x=w901, y=w900) -> (x = y?=w899:bool)
            }
            n364 = case shown="True" w874 {
              tunnel: w879 -> [w894 w898]
              tunnel: [w893 w897] -> w878
              tunnel: w877 -> [w892 w895]
              frame False {
                n365 = call "Connection failed.vi"("error in"=w894, "Connected?"=FALSE, "Module ID"=w892) -> ("error out"=w893:errorcluster)  [unwired: 8 in]
              }
              frame True {
                n366 = call "Device connected.vi"("error in"=w898, "Connected?"=TRUE, "Module ID"=w895) -> ("error out"=w897:errorcluster)  [unwired: 8 in]
              }
            }
            n367 = Bundle By Name(cluster=T32 {"DevSerialNum"=0, "error"={"status"=FALSE, "code"=0, "source"=""}} ("Validate connection (Reply Payload)"), "error"=w878) -> (w883:T32)
            n368 = Merge Errors(w889, w878) -> (w881:errorcluster)
            n369 = case shown="True" w884 {
              tunnel: w885 -> [_ w903]
              tunnel: w883 -> [_ w902]
              frame False {
              }
              frame True {
                n370 = Send Notification(notification=w902, notifier=w903) -> ()  [unwired: 1 in, 2 out]
              }
            }
          }
          frame "Start continous acquisition" {
            # "Request to acquire continuously from DAQ device with a predefined Timeout period."
            n371 = Variant To Data(error in=w920, type=T23 {"Module ID"=-1, "Task list"=enum."All", "Timeout"=0, "Acq type"=enum."Single", "N samples"=0, "Data in"=variant} ("Start continous acquisition Argument"), Variant=w919) -> (data=w917:T23, error out=w911:errorcluster)
            n372 = Unbundle By Name(w917) -> ("Module ID"=w915:i32, "Task list"=w907:T4, "Timeout"=w914:i32, "Acq type"=w913:enum16{"Single", "Multiple"}, "N samples"=w912:i32, "Data in"=w904:variant)
            n373 = case shown="Default" w907 {
              tunnel: w906 -> [w922 w924 w926 w928 w930]
              tunnel: [w921 w923 w925 w927 w929] -> w905
              frame Default {
                n374 = Unbundle By Name(w922) -> ("DO task"=w921:refnum<k21>)
              }
              frame "DO task" {
                n375 = Unbundle By Name(w924) -> ("DO task"=w923:refnum<k21>)
              }
              frame "DI task" {
                n376 = Unbundle By Name(w926) -> ("DI task"=w925:refnum<k21>)
              }
              frame "AO task" {
                n377 = Unbundle By Name(w928) -> ("AO task"=w927:refnum<k21>)
              }
              frame "AI task" {
                n378 = Unbundle By Name(w930) -> ("AI task"=w929:refnum<k21>)
              }
            }
            n379 = Bundle By Name(cluster=T3 {"Module ID"=0, "Task list"=enum."All", "Timeout"=0, "Acq type"=enum."Single", "Data in"=variant, "DAQmx Task"="", "N samples"=0} ("event data"), "DAQmx Task"=w905, "Module ID"=w915, "Task list"=w907, "Timeout"=w914, "Acq type"=w913, "N samples"=w912, "Data in"=w904) -> (w908:T3)
            n380 = call "Wake HL.vi"("error in (no error)"=w911, "event data"=w908, "User events"=w909) -> ("error out"=w910:errorcluster)  [unwired: 8 in]
          }
          frame "Stop continuous acquisition" {
            # "Request to stop continous acquisition made by the HL."
            n381 = Variant To Data(error in=w939, type=T24 {"Module ID"=-1, "Boolean"=FALSE} ("Stop continuous acquisition Argument"), Variant=w937) -> (data=w935:T24, error out=w934:errorcluster)
            n382 = Unbundle By Name(w935) -> ("Boolean"=w931:bool)  [unwired: 1 out]
            n383 = call "Sleep HL -- subVI.vi"("error in (no error)"=w934, "User events"=w932, "event data"=w931) -> ("error out"=w933:errorcluster)  [unwired: 8 in]
          }
        }
        n384 = call-dynamic "Delacor_lib_QMH_Error Handler - Message Handling Loop.vi"("error in"=w463, "Message Queue in"=w453) -> ("dup error in"=w460:errorcluster)  [unwired: 8 in, 1 out]
      }
    }
    frame Error {
      n385 = call "Synchronize Caller Events.vi"("Module Admin"=w947) -> ("Module Admin out"=w946:refnum<class "Delacor_lib_QMH_Cloneable Module Admin.lvclass">)  [unwired: 9 in, 1 out]
      n386 = property class="Mod Admin"(reference=w946) -> ("Accessors:Module ID"=w945:i32)  [unwired: 1 in, 2 out]
      n387 = call-dynamic "Delacor_lib_QMH_Release Message Queue.vi"("error in"=w944, "Message Queue"=w942) -> ("error out"=w943:errorcluster)  [unwired: 9 in]
      n388 = call "Module Name--constant.vi"("Module ID"=w945) -> ("Module Name"=w950:string)  [unwired: 10 in]
      n389 = Format Into String(format string="An error occurred during initialization. %s is no longer running.", w950) -> (resulting string=w948:string)  [unwired: 2 in, 1 out]
      n390 = call "Error Reported.vi"("Additional Information"=w948, "Error"=w943, "Module ID"=w945) -> ()  [unwired: 8 in, 1 out]
    }
  }
  n391 = Unregister For Events(event registration refnum=w4, error in=w1) -> (error out=w3:errorcluster)
  n392 = Merge Errors(w26, w25, w3) -> (w6:errorcluster)
  n393 = call "Destroy user events.vi"("error in (no error)"=w6, "User events"=w7) -> ("error out"=w5:errorcluster)  [unwired: 9 in]
  n394 = call "Close Module.vi"("error in"=w5, "Wait for stop?"=w13, "Module Admin in"=w10) -> ("error out"=w23:errorcluster, "External Launch"=w12:bool, "Module Admin out"=w14:refnum<class "Delacor_lib_QMH_Cloneable Module Admin.lvclass">)  [unwired: 6 in]
  n395 = Unregister For Events(event registration refnum=w18, error in=w23) -> (error out=w22:errorcluster)
  "error out" <- w22
  n396 = local write "Module Admin"(w14) -> ()
  n397 = case "External Launch?" shown="True" w12 {
    tunnel: w22 -> [_ w952]
    frame False {
    }
    frame True {
      n398 = case shown="No Error" w952 {
        frame No Error {
          n399 = invoke class="VI" method="FP.Close"() -> ()  [unwired: 3 in, 3 out]
        }
        frame Error {
          n400 = invoke class="VI" method="FP.Open"("Activate"=TRUE ("Activate?")) -> ()  [unwired: 4 in, 5 out]
        }
      }
    }
  }
